vi "运维调试_总氮.vi"() -> ()   [LabVIEW 2016, in "斯坦道总氮.lvlib"]
uses:
  <vilib>/Utility/miscctls.llb/LVPointTypeDef.ctl
  <vilib>/Utility/config.llb/NI_LVConfig.lvlib
  <vilib>/ptbypt/NI_PtbyPt.lvlib
panel:
  out "固件版本号":string
  in  "定时设置":cluster{"启动":bool, "控制命令":T1, "测量参数":T2}(xcontrol)
  out "单位:":T3(ring)
  out "模块版本号":string
  in  "校准按钮":T4
  out "运行状态":T5 {"数据时间:" format="%<%y/%m/%d %H:%M:%S>T"; "仪器时间:" format="%<%y/%m/%d %H:%M:%S>T"}
  out "一级权限":bool
  out "二级权限":bool
  out "输入密码":u32
  out "布尔":bool
  in  "流程固件":bool
  in  "仪器参数设置":bool
  in  "量程参数读取":T6
  in  "模块启用":bool
  in  "串口设置":bool
  in  "公式一键写入":bool
  in  "流程路径":path=path "C:/Users/STD/Documents/斯坦道流程文件/流程.xml"
  in  "曲线模型":cluster{"X^2":dbl, "X":dbl, "B":dbl, "r^2":dbl}(xcontrol)
  out "字符串":string
  in  "质控参数设置":bool
  in  "自动测试量程配置":T7
  out "温度2":sgl
  out "温度1":sgl
  out "ADC":sgl
  in  "数组":string[](array[string])
  in  "量程切换阈值写入":bool
  in  "量程切换阈值读取":bool
  in  "参数下拉列表":enum16{"总磷", "总氮"}(ring)=enum."总氮"
  in  "量程下拉列表":enum16{"低量程", "高量程"}(ring)
  in  "测量模式下拉列表":enum16{"水样测量", "零点核查", "跨度核查", "标样核查", "加标回收"}(ring)
  in  "公式":cluster{"X^2":dbl, "X":dbl, "b":dbl}
  in  "写公式":bool
  in  "读公式":bool
  in  "返回":bool
  in  "设置":bool
  out "集成报警信息":string
  in  "停止":bool
  in  "手动启动":bool
  in  "单步测试":bool
  out "F3":sgl format="%#.6f"
  out "F2":sgl format="%#.6f"
  out "F1":sgl format="%#.6f"
  out "F0":sgl format="%#.6f"
  out "多列列表框":i32(listbox)
  # "参数设置"
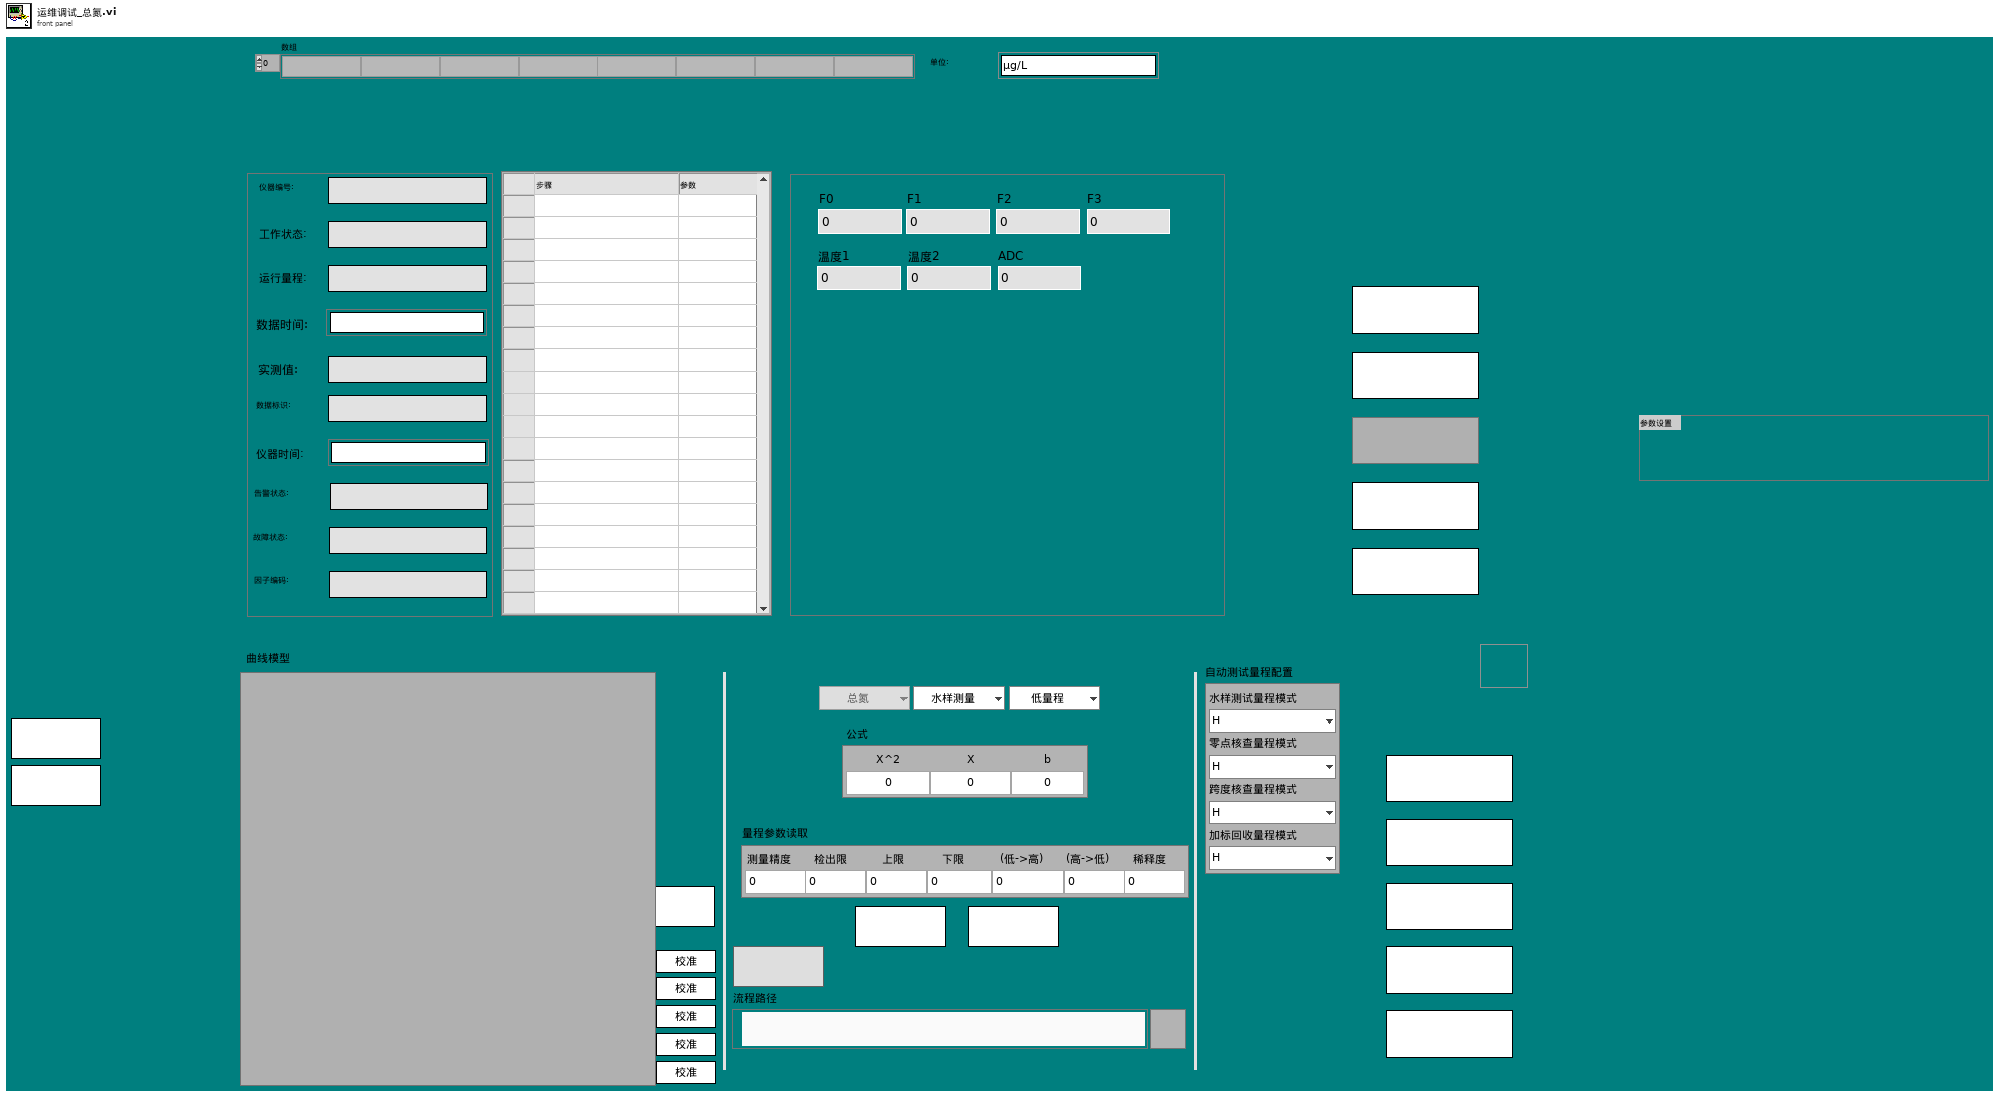
[diagram p1: front panel]
types:
  T1 = typedef "定时设置.xctl/国标控制命令.ctl" = enum16{"启动测量", "标样核查", "零点核查", "跨度核查", "空白测试", "平行样测试", "加标回收", "空白校准", "标样校准", "初始化（清洗）", "停止测试", "仪器重启", "校时", "模式设置", "测量间隔设置"}
  T2 = typedef "定时设置.xctl/测量参数.ctl" = u16
  T3 = enum16{"μg/L", "mg/L", "ppm", "mg/m3", "cm", "ppb", "μg/m3", "%", "nmol/mol", "μmol/mol", "MPN/L", "MPN/100ml", "ng/m3", "NTU", "无量纲", "mS/cm", "μS/cm", "℃", "mV", "cells/mL"}
  T4 = cluster{"校准1":bool, "校准2":bool, "校准3":bool, "校准4":bool, "校准5":bool}
  T5 = cluster{"仪器编号:":string, "工作状态:":string, "运行量程: ":string, "数据时间:":timestamp, "实测值:":string, "数据标识: ":string, "仪器时间:":timestamp, "告警状态: ":string, "故障状态:  ":string, "因子编码:":string}
  T6 = cluster{"测量精度":dbl, "检出限":dbl, "上限":dbl, "下限":dbl, "(低->高)":dbl, "(高->低)":dbl, "稀释度":dbl}
  T7 = cluster{"水样测试量程模式":enum16{"H", "L", "AUTO"}, "空白核查量程模式":enum16{"H", "L", "AUTO"}, "跨度核查量程模式":enum16{"H", "L", "AUTO"}, "加标回收量程模式":enum16{"H", "L", "AUTO"}}
  T8 = typedef "LVPointTypeDef.ctl" = cluster{"Horizontal":i16, "Vertical":i16}
  T9 = cluster{"因子编码":u32, "单位":u16, "标样参考值":sgl, "水样数据时间":timestamp, "水样实测值":sgl, "水样数据标识":string, "标样数据时间":timestamp, "标样实测值":sgl, "标样数据标识":string, "空白数据时间":timestamp, "空白实测值":sgl, "空白数据标识":string, "零点核查数据时间":timestamp, "零点核查实测值":sgl, "零点核查数据标识":string, "跨度核查数据时间":timestamp, "跨度核查实测值":sgl, "跨度核查数据标识":string, "加标回收数据时间":timestamp, "加标回收实测值":sgl, "加标回收数据标识":string, "平行样数据时间":timestamp, "平行样实测值":sgl, "平行样数据标识":string, "F0":sgl, "F1":sgl, "F2":sgl, "F3":sgl, "F4":sgl, "F5":sgl, "F6":sgl, "F7":sgl, "温度":sgl, "湿度":sgl, "X值":sgl, "fidrange":u16}
  T10 = cluster{"系统时间":timestamp, "工作状态":enum16{"空闲", "水样测试", "标样核查", "零点核查", "跨度核查", "空白测试", "平行样测试", "加标回收", "空白校准", "标样校准", "初始化（清洗）"}, "测量模式":enum16{"待机", "连续模式", "周期模式", "定点模式", "受控模式", "手动模式"}, "告警代码":u16, "故障代码":u16, "日志代码":u16, "软件版本":u16, "F0":sgl, "F1":sgl, "F2":sgl, "F3":sgl, "T":sgl, "H":sgl, "id":u16, "flowid":u16, "量程":u16, "总磷控温温度1":sgl, "营养盐控温温度2":sgl, "ADC":sgl}
  T11 = enum16{"空闲", "水样测试", "标样核查", "零点核查", "跨度核查", "空白测试", "平行样测试", "加标回收", "空白校准", "标样校准", "初始化（清洗）"}
  T12 = cluster{"Major":u16, "Minor":u16, "Fix":u16, "Build":u16}
  T13 = typedef "NI_LVConfig.lvlib/Config Data RefNum.ctl" = refnum<k1>
  T14 = cluster{"时间源选择":enum16{"系统时间源", "仪器时间源"}, "外部时间源":timestamp}
  T15 = enum32{"Bad", "Idle", "Run top level", "Running"}
  T16 = enum8{"Enabled", "Disabled", "Disabled and Grayed Out"}
  T17 = cluster{"运行模式":enum16{"维护模式", "常规模式", "应急模式", "质控模式"}, "质控频次":enum16{"关闭", "每天", "星期一", "星期二", "星期三", "星期四", "星期五", "星期六", "星期日"}, "空白核查时间":u16, "跨度核查时间":u16, "24H周期设置":bool[]}
  T18 = cluster{"时间标识":timestamp, "设备":string, "日志信息":string, "备注":string}
  T19 = cluster{"参数":string, "报警内容":string, "报警分析":string}
  T20 = cluster{"启动模式":enum16{"跨度核查", "水样测量", "空白核查", "标样核查", "加标回收"}, "启动参数":u16, "量程":enum16{"低量程", "高量程"}}
  T21 = cluster{"时间标识":timestamp, "设备":string, "日志信息":string, "流程参数":string}
  T22 = typedef "LVRowAndColumnUnsignedTypeDef.ctl" = cluster{"Row":u32, "Column":u32}
  T23 = cluster{"参数下拉列表":enum16{"总磷", "总氮"}, "测量模式下拉列表":enum16{"水样测量", "零点核查", "跨度核查", "标样核查", "加标回收"}, "量程下拉列表":enum16{"低量程", "高量程"}}
  T24 = cluster{"站号":u16, "量程切换":enum32{"H", "L", "AUTO"}, "控制命令":enum16{"启动测量", "标样核查", "零点核查", "跨度核查", "空白测试", "平行样测试", "加标回收", "空白校准", "标样校准", "初始化（清洗）", "停止测试", "仪器重启", "校时", "模式设置", "测量间隔设置"}, "模式设置":enum16{"待机", "连续模式", "周期模式", "定点模式", "受控模式", "手动模式"}, "测量间隔":u16}
  T25 = cluster{"跨度值":dbl, "零点标准液浓度":dbl, "跨度标准液浓度":dbl, "标准液标准浓度":dbl}
  T26 = cluster{"确定":bool, "跨度值":dbl, "零点标准液浓度":dbl, "跨度标准液浓度":dbl, "标准液标准浓度":dbl}
  T27 = cluster{"测量量程":dbl, "测量精度":dbl, "测量间隔":dbl, "消解温度":dbl, "消解时长":dbl, "空白校准时间":timestamp, "曲线截距":dbl, "曲线斜率":dbl, "测量检出限":dbl, "测量信号值":dbl, "线性相关系数":dbl, "二次多项式系数":dbl, "标样校准时间":timestamp, "稀释倍数":dbl, "三项式系数":dbl, "空白标定系数":dbl, "量程系数":dbl, "F0/ORPA":dbl, "F1/ORPB":dbl, "F2/ORPK":dbl, "F3":dbl, "F4":dbl, "F5":dbl, "F6":dbl, "F7":dbl, "X0/滴定数":dbl, "量程":dbl}
  T28 = cluster{"确定":bool, "测量量程":dbl, "测量精度":dbl, "测量间隔":dbl, "消解温度":dbl, "消解时长":dbl, "空白校准时间":timestamp, "曲线截距":dbl, "曲线斜率":dbl, "测量检出限":dbl, "测量信号值":dbl, "线性相关系数":dbl, "二次多项式系数":dbl, "标样校准时间":timestamp, "稀释倍数":dbl, "三项式系数":dbl, "空白标定系数":dbl, "量程系数":dbl, "F0/ORPA":dbl, "F1/ORPB":dbl, "F2/ORPK":dbl, "F3":dbl, "F4":dbl, "F5":dbl, "F6":dbl, "F7":dbl, "X0/滴定数":dbl, "量程":dbl}
  T29 = cluster{"标液浓度1":dbl, "标液浓度2":dbl, "标液浓度3":dbl, "标液浓度4":dbl, "标液浓度5":dbl}
  T30 = cluster{"测量精度":u16, "检出限":dbl, "上限":dbl, "下限":dbl, "阈值（低->高）":dbl, "阈值（高->低）":dbl, "稀释度":dbl}
  T31 = enum16{"Left Button", "Center Button", "Right Button", "Window Close"}
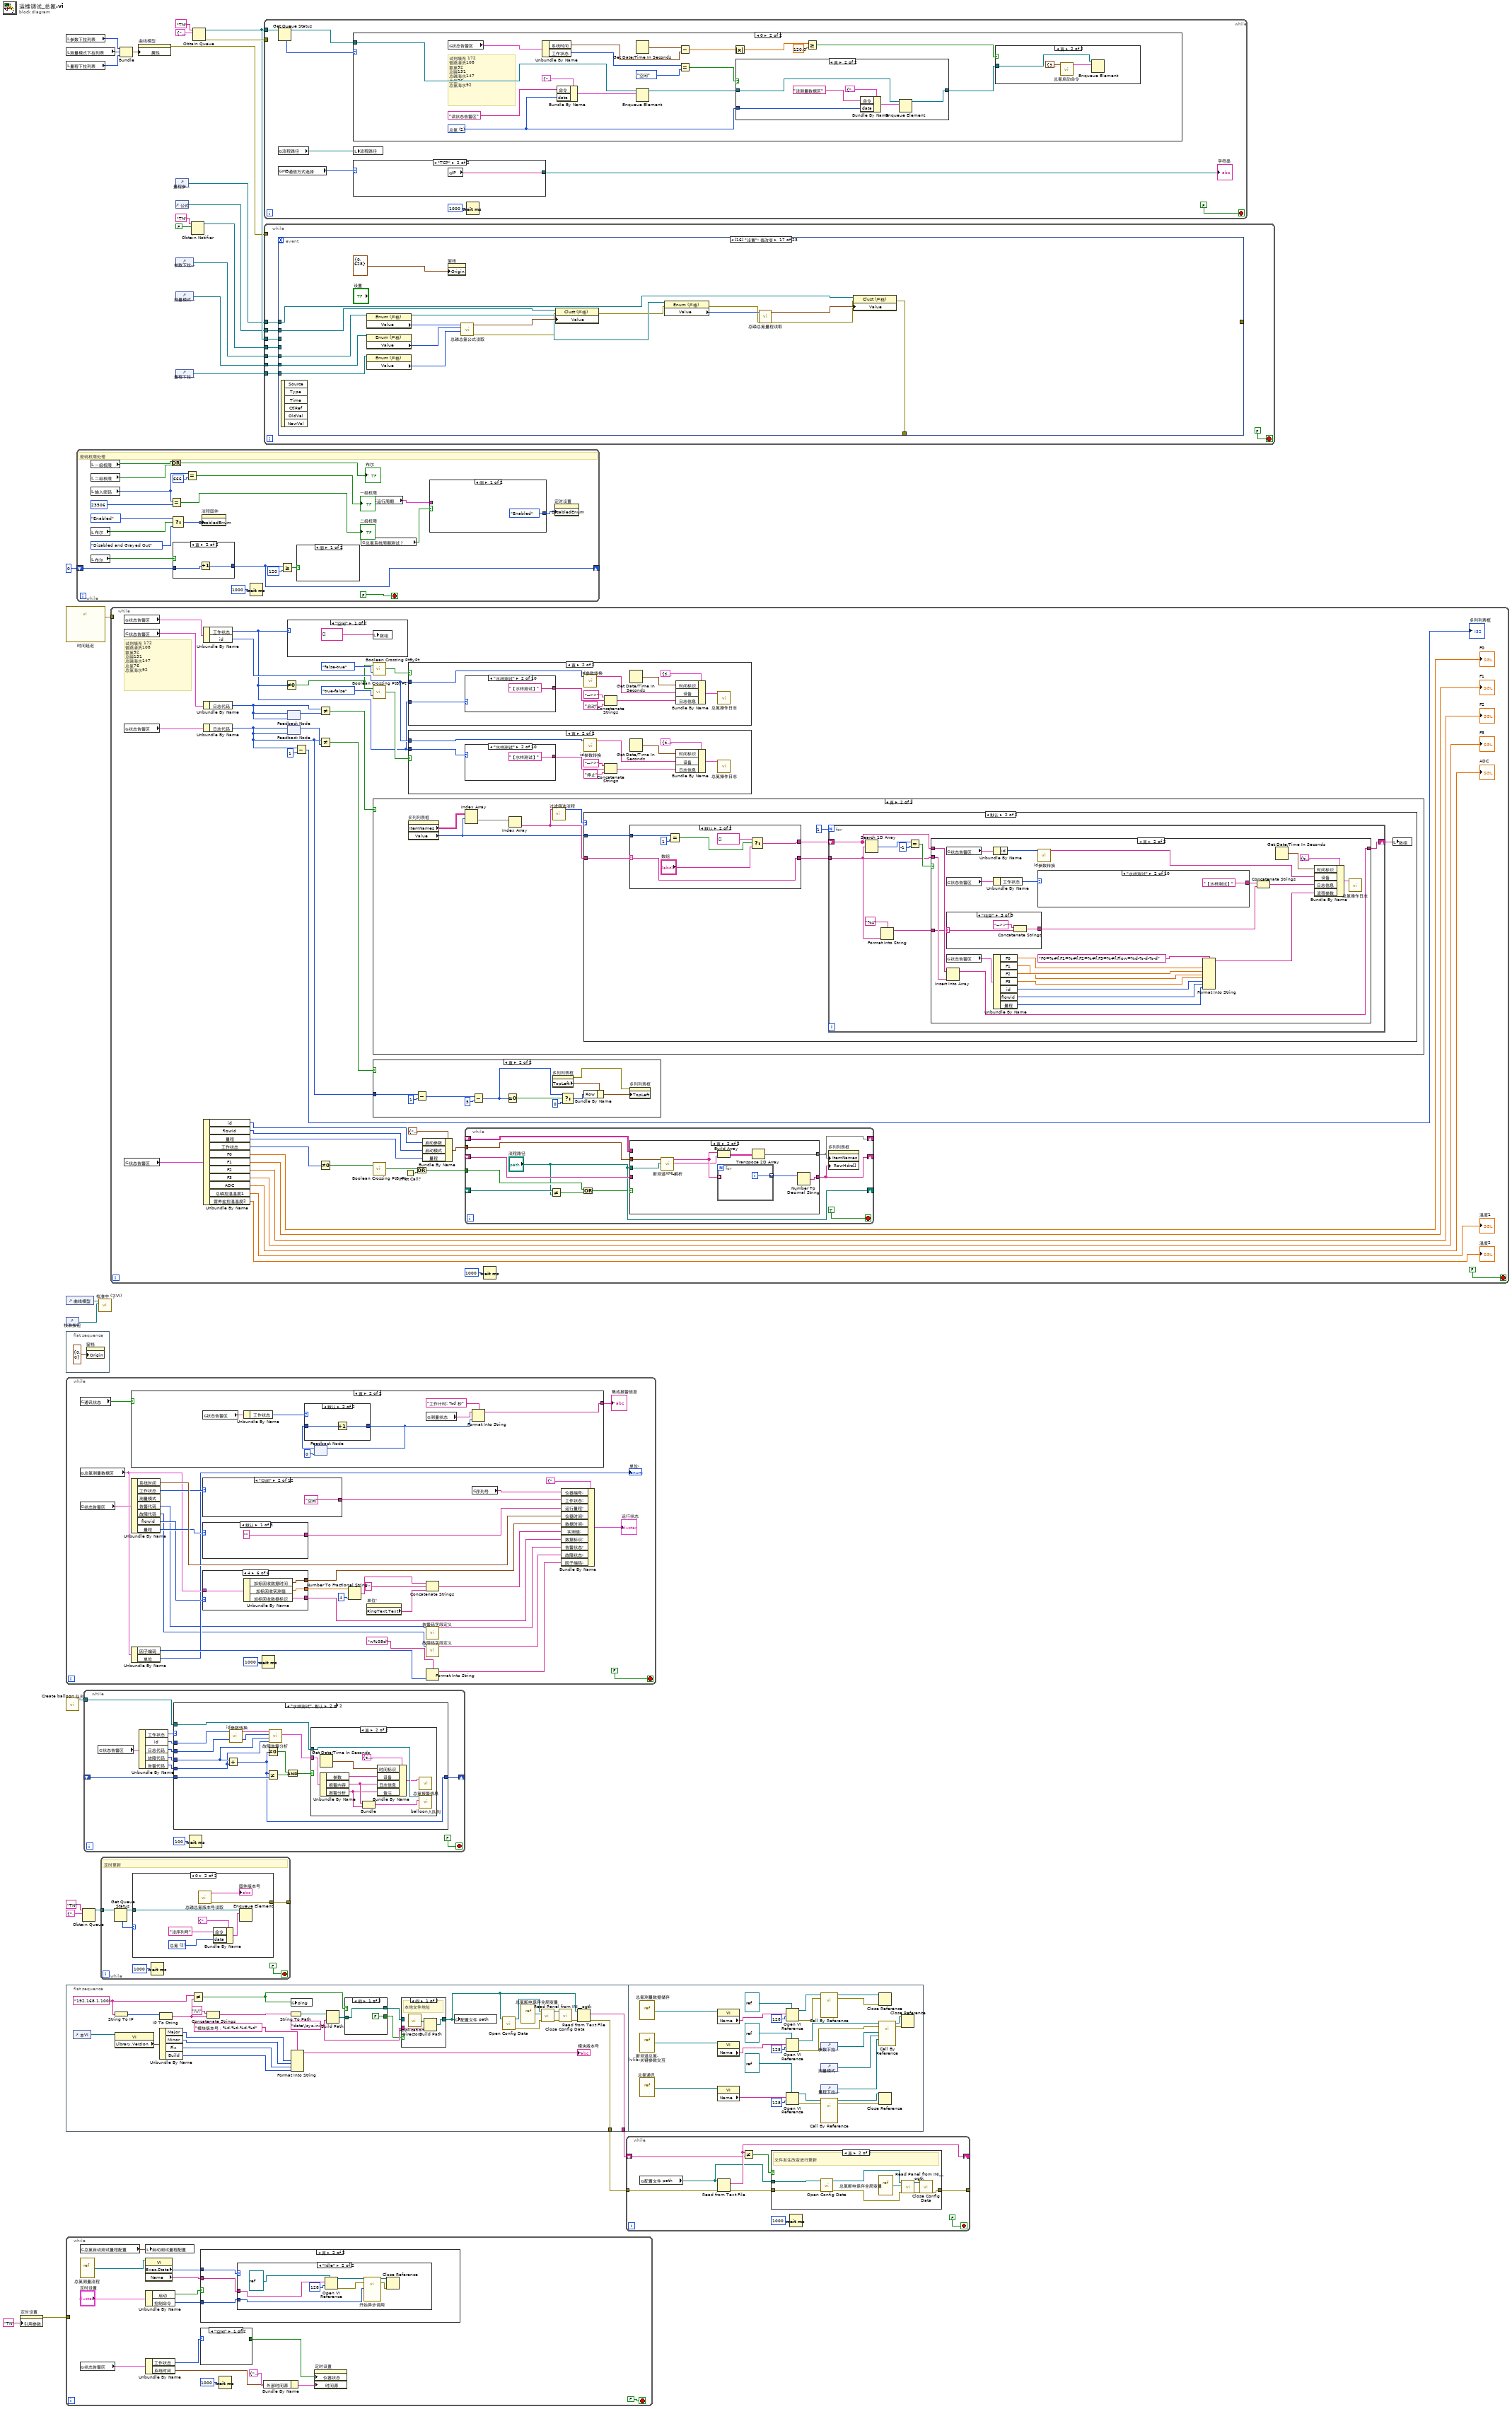
[diagram p0: block diagram]
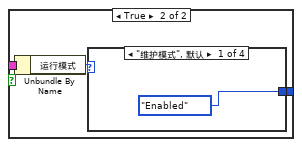
[diagram p5: hidden frame]
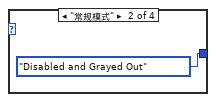
[diagram p6: hidden frame]
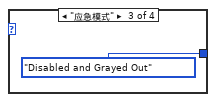
[diagram p7: hidden frame]
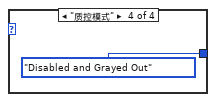
[diagram p8: hidden frame]
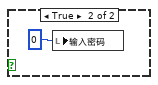
[diagram p9: hidden frame]
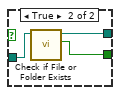
[diagram p11: hidden frame]
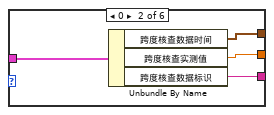
[diagram p15: hidden frame]
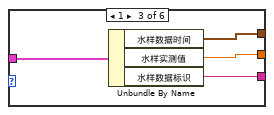
[diagram p16: hidden frame]
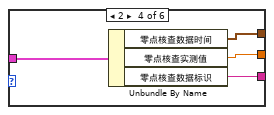
[diagram p17: hidden frame]
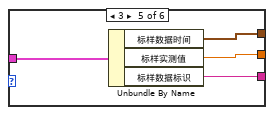
[diagram p18: hidden frame]
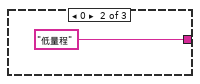
[diagram p19: hidden frame]
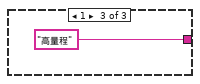
[diagram p20: hidden frame]
diagram:
  n1 = property on="定时设置" class="定时设置 (严格)"("引用参数"="TN") -> (error out=w1:errorcluster)  [unwired: 2 in, 1 out]
  n2 = local read "参数下拉列表"() -> (w12:enum16{"总磷", "总氮"})
  n3 = local read "测量模式下拉列表"() -> (w11:enum16{"水样测量", "零点核查", "跨度核查", "标样核查", "加标回收"})
  n4 = local read "量程下拉列表"() -> (w10:enum16{"低量程", "高量程"})
  n5 = call "时间延迟"() -> ("error out"=w21:errorcluster)  [unwired: 11 in]
  n6 = control-ref of="曲线模型"() -> (w6:refnum<vi>)
  n7 = control-ref of="校准按钮"() -> (w5:refnum<vi>)
  n8 = flat-sequence {
    frame #0 {
      n9 = property on="窗格" class="Pane"("Origin"=T8 {"Horizontal"=0, "Vertical"=0} ("原点")) -> ()  [unwired: 2 in, 2 out]
    }
  }
  n10 = while {
    stop <- FALSE stop-if-true
    n11 = global read "VAR总氮全局变量.vi" "通讯状态"() -> (w59:bool)
    n12 = global read "VAR总氮全局变量.vi" "总氮测量数据区"() -> (w48:T9)
    n13 = global read "VAR总氮全局变量.vi" "状态告警区"() -> (w51:T10)
    n14 = case shown="真" w59 {
      tunnel: ["通讯异常" ("集成报警信息") w102] -> w58
      frame False {
      }
      frame True {
        n15 = global read "VAR总氮全局变量.vi" "状态告警区"() -> (w108:T10)
        n16 = Unbundle By Name(w108) -> ("工作状态"=w107:T11)
        n17 = feedback #1(0) -> (w105:i32)
        n18 = case shown="默认" w107 {
          tunnel: w105 -> [_ w110]
          tunnel: [_ w109] -> w103
          frame "空闲" {
          }
          frame Default {
            n19 = Increment(x=w110) -> (x+1=w109:i32)
          }
        }
        n20 = feedback-in #1(w103) -> ()
        n21 = global read "VAR总氮全局变量.vi" "测量状态"() -> (w101:string)
        n22 = Format Into String(format string="工作计时: %d 秒" ("格式字符串"), initial string=w101, w103) -> (resulting string=w102:string)  [unwired: 1 in, 1 out]
      }
    }
    "集成报警信息" <- w58
    n23 = Unbundle By Name(w51) -> ("系统时间"=w57:timestamp, "工作状态"=w49:T11, "告警代码"=w34:u16, "故障代码"=w32:u16, "flowid"=w47:u16, "量程"=w55:u16)  [unwired: 1 out]
    n24 = Unbundle By Name(w48) -> ("因子编码"=w52:u32, "单位"=→"单位:":u16)
    n25 = case shown="\"空闲\"" w49 {
      selector: w49 -> [w85 _ _ _ _ _ _ _ _ _ _ _]
      tunnel: [w86 "空闲" ("工作状态") "水样测量" ("工作状态") "标样核查" ("工作状态") "零点核查" ("工作状态") "跨度核查" ("工作状态") "空白测试" ("工作状态") "平行样测试" ("工作状态") "加标回收" ("工作状态") "空白校准" ("工作状态") "标样校准" ("工作状态") "初始化" ("工作状态")] -> w56
      frame Default {
        n26 = Format Into String(format string="%d" ("格式字符串"), initial string="未知" ("工作状态"), w85) -> (resulting string=w86:string)  [unwired: 1 in, 1 out]
      }
      frame "空闲" {
      }
      frame "水样测试" {
      }
      frame "标样核查" {
      }
      frame "零点核查" {
      }
      frame "跨度核查" {
      }
      frame "空白测试" {
      }
      frame "平行样测试" {
      }
      frame "加标回收" {
      }
      frame "空白校准" {
      }
      frame "标样校准" {
      }
      frame "初始化（清洗）" {
      }
    }
    n27 = case shown="默认" w55 {
      tunnel: ["" ("字符串") "低量程" ("字符串") "高量程" ("字符串")] -> w54
      frame Default {
      }
      frame 0 {
      }
      frame 1 {
      }
    }
    n28 = case shown="4" w47 {
      tunnel: [_ w65 w69 w73 w77 w81] -> w43
      tunnel: [_ w63 w68 w72 w76 w80] -> w39
      tunnel: [_ w62 w67 w71 w75 w79] -> w36
      tunnel: w48 -> [_ w64 w66 w70 w74 w78]
      frame Default {
      }
      frame 0 {
        n29 = Unbundle By Name(w64) -> ("跨度核查数据时间"=w65:timestamp, "跨度核查实测值"=w63:sgl, "跨度核查数据标识"=w62:string)
      }
      frame 1 {
        n30 = Unbundle By Name(w66) -> ("水样数据时间"=w69:timestamp, "水样实测值"=w68:sgl, "水样数据标识"=w67:string)
      }
      frame 2 {
        n31 = Unbundle By Name(w70) -> ("零点核查数据时间"=w73:timestamp, "零点核查实测值"=w72:sgl, "零点核查数据标识"=w71:string)
      }
      frame 3 {
        n32 = Unbundle By Name(w74) -> ("标样数据时间"=w77:timestamp, "标样实测值"=w76:sgl, "标样数据标识"=w75:string)
      }
      frame 4 {
        n33 = Unbundle By Name(w78) -> ("加标回收数据时间"=w81:timestamp, "加标回收实测值"=w80:sgl, "加标回收数据标识"=w79:string)
      }
    }
    n34 = Wait (ms)(milliseconds to wait=u32 1000 ("等待时间（毫秒）")) -> ()  [unwired: 1 out]
    n35 = Number To Fractional String(number=w39, precision (6)=i16 4 ("精度(6)")) -> (F-format string=w38:string)  [unwired: 2 in]
    n36 = property on="单位:" class="Enum (严格)"() -> ("RingText.Text"=w40:string)  [unwired: 2 in, 2 out]
    n37 = Concatenate Strings(w38, " " ("字符串"), w40) -> (w37:string)
    n38 = call "告警码字段定义.vi"("告警代码"=w34) -> ("字符串"=w33:string)  [unwired: 8 in, 2 out]
    n39 = call "故障码字段定义.vi"("故障代码"=w32) -> ("字符串"=w31:string)  [unwired: 10 in]
    n40 = Format Into String(format string="w%05d" ("格式字符串"), w52) -> (resulting string=w35:string)  [unwired: 2 in, 1 out]
    n41 = global read "VAR总氮全局变量.vi" "序列号"() -> (w50:string)
    n42 = Bundle By Name(cluster=T5 {"仪器编号:"="", "工作状态:"="", "运行量程: "="", "数据时间:"=timestamp(0 s since 1904-01-01), "实测值:"="", "数据标识: "="", "仪器时间:"=timestamp(0 s since 1904-01-01), "告警状态: "="", "故障状态:  "="", "因子编码:"=""} ("运行状态"), "仪器编号:"=w50, "工作状态:"=w56, "运行量程:"=w54, "仪器时间:"=w57, "数据时间:"=w43, "实测值:"=w37, "数据标识:"=w36, "告警状态:"=w33, "故障状态:"=w31, "因子编码:"=w35) -> (→"运行状态":T5)
  }
  n43 = call "Create balloon 队列.vi"() -> ("队列输出"=w3:refnum<queue>)  [unwired: 11 in]
  n44 = flat-sequence {
    tunnel: [w120] -> w4
    tunnel: [w119] -> w7
    frame #0 {
      w133 = "data\\sys.ini" ("名称或相对路径")
      w125 = "192.168.1.100" ("名称")
      n45 = control-ref of="本VI"() -> (w118:refnum<vi>)
      n46 = String To IP(1:w125) -> (0:w132:u32)
      n47 = property class="VI"(reference=w118) -> ("Library.Version"=w117:T12)  [unwired: 1 in, 2 out]
      n48 = IP To String(2:w132) -> (0:w129:string)  [unwired: 1 in]
      n49 = Unbundle By Name(w117) -> ("Major"=w115:u16, "Minor"=w114:u16, "Fix"=w113:u16, "Build"=w112:u16)
      n50 = Not Equal?(x=w125, y=w129) -> (x != y?=w123:bool)
      n51 = Concatenate Strings("\\\\" ("字符串"), w129) -> (w130:string)
      n52 = String To Path(string=w130) -> (path=w124:path)
      n53 = global write "VAR总氮全局变量.vi" "ping"(w123) -> ()
      n54 = Format Into String(format string="模块版本号：%d.%d.%d.%d" ("格式字符串"), w115, w114, w113, w112) -> (resulting string=→"模块版本号":string)  [unwired: 2 in, 1 out]
      n55 = Build Path(base path=w124, name or relative path=w133) -> (appended path=w128:path)
      n56 = case shown="假" w123 {
        tunnel: w128 -> [w139 w143]
        tunnel: [w139 w142] -> w127
        tunnel: [FALSE w141] -> w126
        frame False {
        }
        frame True {
          n57 = call <vilib>:"Check if File or Folder Exists.vi"("path"=w143) -> ("file or folder exists?"=w141:bool, "dup path"=w142:path)  [unwired: 8 in, 1 out]
        }
      }
      n58 = case shown="假" w126 {
        tunnel: w127 -> [_ w147]
        tunnel: [w145 w147] -> w122
        tunnel: w133 -> [w144 _]
        frame False {
          # "本地文件地址"
          n59 = call <vilib>:"Application Directory.vi"() -> ("Application Directory"=w146:path)
          n60 = Build Path(base path=w146, name or relative path=w144) -> (appended path=w145:path)
        }
        frame True {
          # "网络共享地址"
        }
      }
      n61 = global write "VAR总氮全局变量.vi" "配置文件 path"(w122) -> ()
      n62 = call <vilib>:"Open Config Data.vi"("configuration file path"=w122) -> ("error out"=w135:errorcluster, "refnum"=w138:T13)  [unwired: 8 in, 1 out]
      n63 = vi-ref "总氮断电保存全局变量.vi"() -> (w137:refnum<vi>)
      n64 = call <userlib>:"Read Panel from INI__ogtk.vi"("error in (no error)"=w135, "VI ref"=w137, "refnum"=w138) -> ("error out"=w134:errorcluster, "refnum out"=w136:T13)  [unwired: 7 in]
      n65 = call <vilib>:"Close Config Data.vi"("error in (no error)"=w134, "refnum"=w136) -> ("error out"=w121:errorcluster)  [unwired: 8 in, 1 out]
      n66 = Read from Text File(file (use dialog)=w122, error in=w121) -> (text=w119:string, error out=w120:errorcluster)  [unwired: 2 in, 2 out]
    }
    frame #1 {
      n67 = vi-ref "总氮测量数据储存.vi"() -> (w166:refnum<vi>)
      n68 = vi-ref "斯坦道总氮.lvlib:关键参数交互.vi"() -> (w151:refnum<vi>)
      n69 = vi-ref "总氮通讯.vi"() -> (w174:refnum<vi>)
      n70 = property class="VI"(reference=w166) -> ("Name"=w159:string)  [unwired: 1 in, 2 out]
      n71 = property class="VI"(reference=w151) -> ("Name"=w158:string)  [unwired: 1 in, 2 out]
      n72 = property class="VI"(reference=w174) -> ("Name"=w173:string)  [unwired: 1 in, 2 out]
      n73 = Open VI Reference(type specifier VI Refnum (for type only)=refnum<vi> refnum, vi path=w159, options=128 ("选项")) -> (vi reference=w161:refnum<vi>, error out=w163:errorcluster)  [unwired: 3 in]
      n74 = Open VI Reference(type specifier VI Refnum (for type only)=refnum<vi> refnum, vi path=w158, options=128 ("选项")) -> (vi reference=w156:refnum<vi>, error out=w154:errorcluster)  [unwired: 3 in]
      n75 = Open VI Reference(type specifier VI Refnum (for type only)=refnum<vi> refnum, vi path=w173, options=128 ("选项")) -> (vi reference=w171:refnum<vi>, error out=w169:errorcluster)  [unwired: 3 in]
      n76 = call-by-ref "?"(reference=w161, error in=w163) -> (reference out=w165:refnum<vi>, error out=w164:errorcluster)  [unwired: 12 in]
      n77 = control-ref of="参数下拉列表"() -> (w150:refnum<vi>)
      n78 = control-ref of="测量模式下拉列表"() -> (w149:refnum<vi>)
      n79 = control-ref of="量程下拉列表"() -> (w148:refnum<vi>)
      n80 = call-by-ref "?"(reference=w171, error in=w169) -> (reference out=w167:refnum<vi>, error out=w168:errorcluster)  [unwired: 12 in]
      n81 = Close Reference(reference=w165, error in (no error)=w164) -> ()  [unwired: 1 out]
      n82 = call-by-ref "?"(reference=w156, error in=w154, "量程下拉列表"=w148, "测量模式下拉列表"=w149, "测量参数"=w150) -> (reference out=w152:refnum<vi>, error out=w153:errorcluster)  [unwired: 9 in]
      n83 = Close Reference(reference=w167, error in (no error)=w168) -> ()  [unwired: 1 out]
      n84 = Close Reference(reference=w152, error in (no error)=w153) -> ()  [unwired: 1 out]
    }
  }
  n85 = while {
    tunnel: w1 -> [_]
    stop <- FALSE stop-if-true
    n86 = global read "总氮断电保存全局变量.vi" "总氮自动测试量程配置"() -> (w187:T7)
    n87 = vi-ref "总氮测量流程.vi"() -> (w186:refnum<vi>)
    n88 = global read "VAR总氮全局变量.vi" "状态告警区"() -> (w180:T10)
    n89 = local write "自动测试量程配置"(w187) -> ()
    n90 = property class="VI"(reference=w186) -> ("Exec.State"=w184:T15, "Name"=w185:string)  [unwired: 1 in, 2 out]
    n91 = Unbundle By Name("定时设置") -> ("启动"=w181:bool, "控制命令"=w182:T1)
    n92 = Unbundle By Name(w180) -> ("工作状态"=w179:T11, "系统时间"=w175:timestamp)
    n93 = case shown="真" w181 {
      tunnel: w185 -> [_ w193]
      tunnel: w182 -> [_ w192]
      tunnel: w184 -> [_ w191]
      frame False {
      }
      frame True {
        n94 = case shown="\"Idle\"" w191 {
          tunnel: w193 -> [_ w197]
          tunnel: w192 -> [_ w195]
          frame "Bad", Default {
          }
          frame "Idle" {
            n95 = Open VI Reference(type specifier VI Refnum (for type only)=refnum<vi> refnum, vi path=w197, options=128 ("选项")) -> (vi reference=w198:refnum<vi>, error out=w199:errorcluster)  [unwired: 3 in]
            n96 = call-by-ref "开始异步调用"(reference=w198, error in=w199, "控制命令"=w195) -> (reference out=w200:refnum<vi>, error out=w201:errorcluster)  [unwired: 11 in]
            n97 = Close Reference(reference=w200, error in (no error)=w201) -> ()  [unwired: 1 out]
          }
        }
      }
    }
    n98 = case shown="\"空闲\"" w179 {
      tunnel: [_ TRUE] -> w178
      frame "空闲" {
      }
      frame "水样测试", Default {
      }
    }
    n99 = Wait (ms)(milliseconds to wait=u32 1000 ("等待时间（毫秒）")) -> ()  [unwired: 1 out]
    n100 = Bundle By Name(cluster=T14 {"时间源选择"=enum."仪器时间源", "外部时间源"=timestamp(0 s since 1904-01-01)} ("时间源"), "外部时间源"=w175) -> (w176:T14)
    n101 = property on="定时设置" class="定时设置 (严格)"("仪器状态"=w178, "时间源"=w176) -> ()  [unwired: 2 in, 2 out]
  }
  n102 = while {
    shift-right: [w211] -> _
    shift-left: u32 0 ("等待时间（毫秒）") -> [w212]
    stop <- FALSE stop-if-true
    # "密码权限处理"
    n103 = local read "一级权限"() -> (w215:bool)
    n104 = local read "二级权限"() -> (w216:bool)
    n105 = local read "输入密码"() -> (w219:u32)
    n106 = local read "布尔"() -> (w208:bool)
    n107 = local read "布尔"() -> (w213:bool)
    n108 = Or(x=w215, y=w216) -> (x .or. y?=→"布尔":bool)
    n109 = Equal?(x=w219, y=u32 23506) -> (x = y?=→"二级权限":bool)
    n110 = Select(t=T16."Enabled" ("禁用"), s=w208, f=T16."Disabled and Grayed Out") -> (s? t:f=w206:T16)
    n111 = case shown="真" w213 {
      tunnel: w212 -> [_ w234]
      tunnel: [_ w233] -> w211
      frame False {
      }
      frame True {
        n112 = Increment(x=w234) -> (x+1=w233:u32)
      }
    }
    n113 = Equal?(x=w219, y=u32 666) -> (x = y?=→"一级权限":bool)
    n114 = property on="流程固件" class="Bool"("DisabledEnum"=w206) -> ()  [unwired: 2 in, 2 out]
    n115 = Wait (ms)(milliseconds to wait=u32 1000 ("等待时间（毫秒）")) -> ()  [unwired: 1 out]
    n116 = Greater Or Equal?(x=w211, y=u32 120) -> (x >= y?=w209:bool)
    n117 = case shown="假" w209 {
      frame False {
      }
      frame True {
        n118 = local write "输入密码"(u32 0 ("输入密码")) -> ()
      }
    }
    n119 = global read "总氮断电保存全局变量.vi" "总氮系统周期测试？"() -> (w203:bool)
    n120 = global read "总氮断电保存全局变量.vi" "运行周期"() -> (w204:T17)
    n121 = case shown="假" w203 {
      tunnel: w204 -> [_ w227]
      tunnel: [T16."Enabled" ("禁用") w225] -> w202
      frame False {
      }
      frame True {
        n122 = Unbundle By Name(w227) -> ("运行模式"=w226:enum16{"维护模式", "常规模式", "应急模式", "质控模式"})
        n123 = case shown="\"维护模式\", 默认" w226 {
          tunnel: [T16."Enabled" ("禁用") T16."Disabled and Grayed Out" ("禁用") T16."Disabled and Grayed Out" ("禁用") T16."Disabled and Grayed Out" ("禁用")] -> w225
          frame "维护模式", Default {
          }
          frame "常规模式" {
          }
          frame "应急模式" {
          }
          frame "质控模式" {
          }
        }
      }
    }
    n124 = property on="定时设置" class="定时设置 (严格)"("DisabledEnum"=w202) -> ()  [unwired: 2 in, 2 out]
  }
  n125 = Obtain Queue(name (unnamed)="TN" ("名称（未命名）"), element data type=cluster{"命令":string, "data":variant} {"命令"="", "data"=variant}) -> (queue out=w18:refnum<queue>)  [unwired: 3 in, 2 out]
  n126 = while {
    tunnel: w3 -> [w241]
    shift-right: [w237] -> _
    shift-left: _ -> [w238]
    stop <- FALSE stop-if-true
    n127 = global read "VAR总氮全局变量.vi" "状态告警区"() -> (w235:T10)
    n128 = Unbundle By Name(w235) -> ("工作状态"=w236:T11, "id"=w243:u16, "日志代码"=w242:u16, "故障代码"=w240:u16, "告警代码"=w239:u16)
    n129 = case shown="\"水样测试\", 默认" w236 {
      tunnel: w243 -> [_ w258]
      tunnel: w242 -> [_ w257]
      tunnel: w241 -> [_ w254]
      tunnel: w240 -> [_ w253]
      tunnel: w239 -> [_ w252]
      tunnel: w238 -> [w246 w251]
      tunnel: [w246 w250] -> w237
      frame "空闲" {
      }
      frame "水样测试", Default {
        n130 = Add(x=w253, y=w252) -> (x+y=w250:u16)
        n131 = call "id参数转换.vi"("id"=w258) -> ("table输出"=w255:string)  [unwired: 10 in]
        n132 = Not Equal To 0?(x=w250) -> (x != 0?=w249:bool)
        n133 = Not Equal?(x=w250, y=w251) -> (x != y?=w248:bool)
        n134 = call "故障告警分析.vi"("告警代码"=w252, "故障代码"=w253, "运行步序"=w257, "参数"=w255) -> ("报警内容"=w256:T19)  [unwired: 6 in, 1 out]
        n135 = And(x=w249, y=w248) -> (x .and. y?=w247:bool)
        n136 = case shown="真" w247 {
          tunnel: w256 -> [_ w267]
          tunnel: w254 -> [_ w266]
          frame False {
          }
          frame True {
            n137 = Get Date/Time In Seconds() -> (seconds since 1Jan1904=w265:timestamp)
            n138 = Unbundle By Name(w267) -> ("参数"=w262:string, "报警内容"=w261:string, "报警分析"=w260:string)
            n139 = Bundle("报警内容"=w261, "报警分析"=w260) -> (w259:cluster{"报警内容":string, "报警分析":string})  [unwired: 1 in]
            n140 = Bundle By Name(cluster=T18 {"时间标识"=timestamp(0 s since 1904-01-01), "设备"="", "日志信息"="", "备注"=""} ("data in"), "时间标识"=w265, "设备"=w262, "日志信息"=w261, "备注"=w260) -> (w264:T18)
            n141 = call "总氮报警信息.vi"("data in"=w264) -> ()  [unwired: 10 in, 1 out]
            n142 = call "balloon入队列.vi"("报警内容"=w259, "队列"=w266) -> ()  [unwired: 9 in, 1 out]
          }
        }
      }
    }
    n143 = Wait (ms)(milliseconds to wait=u32 100) -> ()  [unwired: 1 out]
  }
  n144 = call "校准中 (子VI).vi"("曲线模型"=w6, "校准按钮"=w5) -> ()  [unwired: 9 in]
  n145 = while {
    tunnel: w18 -> [w272]
    tunnel: [w270] -> _
    stop <- FALSE stop-if-true
    # "定时更新"
    n146 = Get Queue Status(queue=w272) -> (queue out=w269:refnum<queue>, # elements in queue=w268:i32)  [unwired: 2 in, 6 out]
    n147 = case shown="0" w268 {
      tunnel: [_ w276] -> w270
      tunnel: w269 -> [_ w275]
      frame Default {
      }
      frame 0 {
        w278 = u16 2 items=["总磷"=1, "总氮"=2, "氨氮"=3] ("站号")
        n148 = call "总磷总氮版本号读取.vi"() -> ("error out"=w276:errorcluster, "固件版本号"=→"固件版本号":string)  [unwired: 10 in]
        n149 = Bundle By Name(cluster=cluster{"命令":string, "data":variant} {"命令"="", "data"=variant} ("元素"), "命令"="读序列号", "data"=w278) -> (w277:cluster{"命令":string, "data":variant})
        n150 = Enqueue Element(queue=w275, element=w277) -> ()  [unwired: 2 in, 3 out]
      }
    }
    n151 = Wait (ms)(milliseconds to wait=u32 1000 ("等待时间（毫秒）")) -> ()  [unwired: 1 out]
  }
  n152 = while {
    tunnel: w21 -> [_]
    stop <- FALSE stop-if-true
    # "试剂填充 172 \n管路清洗108\n氨氮92\n总磷131\n总磷海水147\n总氮76\n总氮海水92"
    n153 = global read "VAR总氮全局变量.vi" "状态告警区"() -> (w301:T10)
    n154 = global read "VAR总氮全局变量.vi" "状态告警区"() -> (w299:T10)
    n155 = global read "VAR总氮全局变量.vi" "状态告警区"() -> (w303:T10)
    n156 = global read "VAR总氮全局变量.vi" "状态告警区"() -> (w311:T10)
    n157 = Unbundle By Name(w301) -> ("工作状态"=w281:T11, "id"=w285:u16)
    n158 = Unbundle By Name(w299) -> ("日志代码"=w298:u16)
    n159 = Unbundle By Name(w303) -> ("日志代码"=w295:u16)
    n160 = Unbundle By Name(w311) -> ("id"=w308:u16, "flowid"=w310:u16, "量程"=w309:u16, "工作状态"=w289:T11, "F0"=→"F0":sgl, "F1"=→"F1":sgl, "F2"=→"F2":sgl, "F3"=→"F3":sgl, "ADC"=→"ADC":sgl, "总磷控温温度1"=→"温度1":sgl, "营养盐控温温度2"=→"温度2":sgl)
    n161 = Not Equal To 0?(x=w281) -> (x != 0?=w283:bool)
    n162 = case shown="\"空闲\"" w281 {
      frame "空闲" {
        n163 = local write "数组"(string[] [] ("数组")) -> ()
      }
      frame "水样测试", Default {
      }
    }
    n164 = feedback #2(w298) -> (w300:u16)
    n165 = feedback-in #2(w298) -> ()
    n166 = feedback-in #3(w295) -> ()
    n167 = feedback #3(w295) -> (w316:u16)
    n168 = Subtract(x=w295, y=1) -> (x-y=→"多列列表框":i32)
    n169 = Not Equal?(x=w298, y=w300) -> (x != y?=w297:bool)
    n170 = Not Equal?(x=w295, y=w316) -> (x != y?=w315:bool)
    n171 = Not Equal To 0?(x=w289) -> (x != 0?=w313:bool)
    n172 = call <vilib>:"Boolean Crossing PtByPt.vi"("direction"=enum16{"either", "false-true", "true-false"}."false-true", "input"=w283) -> ("crossing"=w287:bool)  [unwired: 1 in]
    n173 = call <vilib>:"Boolean Crossing PtByPt.vi"("direction"=enum16{"either", "false-true", "true-false"}."true-false", "input"=w283) -> ("crossing"=w282:bool)  [unwired: 1 in]
    n174 = case shown="真" w297 {
      frame False {
      }
      frame True {
        n175 = property on="多列列表框" class="MCListbox (严格)"() -> ("ItemNames"=w362:string[][], "Value"=w358:i32)  [unwired: 2 in, 2 out]
        n176 = Index Array(array=w362, index (row)=w358) -> (element=w361:string[])  [unwired: 1 in]
        n177 = Index Array(array=w361) -> (element=w360:string)  [unwired: 1 in]
        n178 = call "过滤筛选流程.vi"("字符串"=w360) -> ("匹配后偏移量"=w359:i32)  [unwired: 10 in]
        n179 = case shown="默认" w359 {
          tunnel: w360 -> [_ w364]
          tunnel: w358 -> [_ w363]
          frame -1 {
          }
          frame Default {
            n180 = case shown="默认" w364 {
              selector: w364 -> [w370 w377]
              tunnel: [w370 w377] -> w366
              tunnel: [string[] [] ("数组") w372] -> w365
              tunnel: w363 -> [_ w376]
              frame "读数" {
              }
              frame Default {
                n181 = Equal?(x=w376, y=1) -> (x = y?=w374:bool)
                n182 = Select(t=string[] [], s=w374, f="数组") -> (s? t:f=w372:string[])
              }
            }
            n183 = for {
              N: 1 -> [_]
              tunnel: w366 -> [w379]
              shift-right: [w378] -> w367
              shift-left: w365 -> [w380]
              n184 = Search 1D Array(1D array=w380, element=w379) -> (index of element=w383:i32)  [unwired: 1 in]
              n185 = Format Into String(format string="%s" ("格式字符串"), w379) -> (resulting string=w384:string)  [unwired: 2 in, 1 out]
              n186 = Equal?(x=w383, y=-1) -> (x = y?=w381:bool)
              n187 = case shown="真" w381 {
                tunnel: w384 -> [_ w394]
                tunnel: w380 -> [w386 w398]
                tunnel: w379 -> [_ w397]
                tunnel: [w386 w396] -> w378
                frame False {
                }
                frame True {
                  n188 = global read "VAR总氮全局变量.vi" "状态告警区"() -> (w411:T10)
                  n189 = global read "VAR总氮全局变量.vi" "状态告警区"() -> (w393:T10)
                  n190 = case shown="\"结束\"" w394 {
                    selector: w394 -> [w421 w424 w427]
                    tunnel: [w421 w423 w426] -> w390
                    frame Default {
                    }
                    frame "初始化" {
                      n191 = Concatenate Strings("-->>" ("字符串"), w424) -> (w423:string)
                    }
                    frame "结束" {
                      n192 = Concatenate Strings("-->>" ("字符串"), w427) -> (w426:string)
                    }
                  }
                  n193 = global read "VAR总氮全局变量.vi" "状态告警区"() -> (w408:T10)
                  n194 = Insert Into Array(array=w398, new element=w397) -> (w396:string[])  [unwired: 1 in]
                  n195 = Unbundle By Name(w411) -> ("id"=w388:u16)
                  n196 = Unbundle By Name(w393) -> ("工作状态"=w392:T11)
                  n197 = Unbundle By Name(w408) -> ("F0"=w405:sgl, "F1"=w404:sgl, "F2"=w403:sgl, "F3"=w402:sgl, "id"=w401:u16, "flowid"=w400:u16, "量程"=w399:u16)
                  n198 = call "id参数转换.vi"("id"=w388) -> ("table输出"=w387:string)  [unwired: 10 in]
                  n199 = case shown="\"水样测试\"" w392 {
                    tunnel: [_ "【水样测试】" ("字符串") "【标样核查】" ("字符串") "【零点核查】" ("字符串") "【跨度核查】" ("字符串") "【空白测试】" ("字符串") "【平行样测试】" ("字符串") "【加标回收】" ("字符串") "【空白校准】" ("字符串") "【标样校准】" ("字符串")] -> w391
                    frame "空闲", Default {
                    }
                    frame "水样测试" {
                    }
                    frame "标样核查" {
                    }
                    frame "零点核查" {
                    }
                    frame "跨度核查" {
                    }
                    frame "空白测试" {
                    }
                    frame "平行样测试" {
                    }
                    frame "加标回收" {
                    }
                    frame "空白校准" {
                    }
                    frame "标样校准" {
                    }
                  }
                  n200 = Format Into String(format string="F0=%#f,F1=%#f,F2=%#f,F3=%#f,Flow=%d-%-d-%-d" ("格式字符串"), w405, w404, w403, w402, w401, w400, w399) -> (resulting string=w406:string)  [unwired: 2 in, 1 out]
                  n201 = Concatenate Strings(w391, w390) -> (w389:string)
                  n202 = Get Date/Time In Seconds() -> (seconds since 1Jan1904=w409:timestamp)
                  n203 = Bundle By Name(cluster=T21 {"时间标识"=timestamp(0 s since 1904-01-01), "设备"="", "日志信息"="", "流程参数"=""} ("data in"), "时间标识"=w409, "设备"=w387, "日志信息"=w389, "流程参数"=w406) -> (w410:T21)
                  n204 = call "总氮操作日志.vi"("data in"=w410) -> ()  [unwired: 11 in]
                }
              }
            }
            n205 = local write "数组"(w367) -> ()
          }
        }
      }
    }
    n206 = case shown="真" w315 {
      tunnel: w295 -> [_ w452]
      frame False {
      }
      frame True {
        n207 = Subtract(x=w452, y=1) -> (x-y=w450:i32)
        n208 = Subtract(x=w450, y=5) -> (x-y=w454:i32)
        n209 = Greater Or Equal To 0?(x=w454) -> (x >= 0?=w453:bool)
        n210 = property on="多列列表框" class="MCListbox (严格)"() -> (error out=w458:errorcluster, "TopLeft"=w459:T22)  [unwired: 2 in, 1 out]
        n211 = Select(t=w454, s=w453, f=0) -> (s? t:f=w455:i32)
        n212 = Bundle By Name(cluster=w459, "Row"=w455) -> (w460:T22)
        n213 = property on="多列列表框" class="MCListbox (严格)"(error in=w458, "TopLeft"=w460) -> ()  [unwired: 1 in, 2 out]
      }
    }
    n214 = call <vilib>:"Boolean Crossing PtByPt.vi"("input"=w313) -> ("crossing"=w288:bool)  [unwired: 2 in]
    n215 = First Call?() -> (First Call?: T/F=w314:bool)
    n216 = case shown="真" w287 {
      tunnel: w285 -> [_ w338]
      tunnel: w281 -> [_ w342]
      frame False {
      }
      frame True {
        n217 = case shown="\"水样测试\"" w342 {
          tunnel: [_ "【水样测试】" ("字符串") "【标样核查】" ("字符串") "【零点核查】" ("字符串") "【跨度核查】" ("字符串") "【空白测试】" ("字符串") "【平行样测试】" ("字符串") "【加标回收】" ("字符串") "【空白校准】" ("字符串") "【标样校准】" ("字符串")] -> w346
          frame "空闲", Default {
          }
          frame "水样测试" {
          }
          frame "标样核查" {
          }
          frame "零点核查" {
          }
          frame "跨度核查" {
          }
          frame "空白测试" {
          }
          frame "平行样测试" {
          }
          frame "加标回收" {
          }
          frame "空白校准" {
          }
          frame "标样校准" {
          }
        }
        n218 = call "id参数转换.vi"("id"=w338) -> ("table输出"=w339:string)  [unwired: 10 in]
        n219 = Concatenate Strings("-->>" ("字符串"), w346, "启动" ("字符串")) -> (w347:string)
        n220 = Get Date/Time In Seconds() -> (seconds since 1Jan1904=w344:timestamp)
        n221 = Bundle By Name(cluster=T21 {"时间标识"=timestamp(0 s since 1904-01-01), "设备"="", "日志信息"="", "流程参数"=""} ("data in"), "时间标识"=w344, "设备"=w339, "日志信息"=w347) -> (w343:T21)
        n222 = call "总氮操作日志.vi"("data in"=w343) -> ()  [unwired: 11 in]
      }
    }
    n223 = case shown="真" w282 {
      tunnel: w285 -> [_ w319]
      tunnel: w281 -> [_ w323]
      frame False {
      }
      frame True {
        n224 = case shown="\"水样测试\"" w323 {
          tunnel: [_ "【水样测试】" ("字符串") "【标样核查】" ("字符串") "【零点核查】" ("字符串") "【跨度核查】" ("字符串") "【空白测试】" ("字符串") "【平行样测试】" ("字符串") "【加标回收】" ("字符串") "【空白校准】" ("字符串") "【标样校准】" ("字符串")] -> w327
          frame "空闲", Default {
          }
          frame "水样测试" {
          }
          frame "标样核查" {
          }
          frame "零点核查" {
          }
          frame "跨度核查" {
          }
          frame "空白测试" {
          }
          frame "平行样测试" {
          }
          frame "加标回收" {
          }
          frame "空白校准" {
          }
          frame "标样校准" {
          }
        }
        n225 = call "id参数转换.vi"("id"=w319) -> ("table输出"=w320:string)  [unwired: 10 in]
        n226 = Concatenate Strings("-->>" ("字符串"), w327, "停止" ("字符串")) -> (w328:string)
        n227 = Get Date/Time In Seconds() -> (seconds since 1Jan1904=w325:timestamp)
        n228 = Bundle By Name(cluster=T21 {"时间标识"=timestamp(0 s since 1904-01-01), "设备"="", "日志信息"="", "流程参数"=""} ("data in"), "时间标识"=w325, "设备"=w320, "日志信息"=w328) -> (w324:T21)
        n229 = call "总氮操作日志.vi"("data in"=w324) -> ()  [unwired: 11 in]
      }
    }
    n230 = Or(x=w288, y=w314) -> (x .or. y?=w312:bool)
    n231 = Bundle By Name(cluster=T20 {"启动模式"=enum."跨度核查", "启动参数"=1, "量程"=enum."低量程"} ("参数簇"), "启动参数"=w308, "启动模式"=w310, "量程"=w309) -> (w302:T20)
    n232 = while {
      tunnel: w312 -> [w438]
      tunnel: w302 -> [w437]
      shift-right: [w432] -> _
      shift-left: _ -> [w434]
      shift-right: [w433] -> _
      shift-left: _ -> [w435]
      shift-right: ["流程路径"] -> _
      shift-left: _ -> [w431]
      stop <- TRUE stop-if-true
      n233 = Not Equal?(x=w431, y="流程路径") -> (x != y?=w428:bool)
      n234 = Or(x=w438, y=w428) -> (x .or. y?=w429:bool)
      n235 = case shown="真" w429 {
        tunnel: [w440 w448] -> w433
        tunnel: [w439 w447] -> w432
        tunnel: w437 -> [_ w442]
        tunnel: w435 -> [w440 _]
        tunnel: w434 -> [w439 _]
        tunnel: "流程路径" -> [_ w441]
        frame False {
        }
        frame True {
          n236 = call "斯坦道XML解析.vi"("添加的路径"=w441, "参数簇"=w442) -> ("步骤时间"=w443:string[], "步骤名"=w445:string[])  [unwired: 8 in]
          n237 = Build Array(w445, w443) -> (w444:string[][])
          n238 = for {
            tunnel: w445 -> [_] mode=indexing
            tunnel: [w449] -> w446 mode=indexing
            i -> [w449]
          }
          n239 = Transpose 2D Array(2D array=w444) -> (transposed array=w447:string[][])
          n240 = Number To Decimal String(number=w446) -> (decimal integer string=w448:string[])  [unwired: 1 in]
        }
      }
      n241 = property on="多列列表框" class="MCListbox (严格)"("ItemNames"=w432, "RowHdrs[]"=w433) -> ()  [unwired: 2 in, 2 out]
    }
    n242 = Wait (ms)(milliseconds to wait=u32 1000 ("等待时间（毫秒）")) -> ()  [unwired: 1 out]
  }
  n243 = Bundle("参数下拉列表"=w12, "测量模式下拉列表"=w11, "量程下拉列表"=w10) -> (w9:T23)  [unwired: 1 in]
  n244 = property on="曲线模型" class="曲线模型 (严格)"("属性"=w9) -> (error out=w17:errorcluster)  [unwired: 2 in, 1 out]
  n245 = control-ref of="量程参数读取"() -> (w13:refnum<vi>)
  n246 = control-ref of="公式"() -> (w22:refnum<vi>)
  n247 = control-ref of="参数下拉列表"() -> (w24:refnum<vi>)
  n248 = control-ref of="测量模式下拉列表"() -> (w23:refnum<vi>)
  n249 = control-ref of="量程下拉列表"() -> (w25:refnum<vi>)
  n250 = Obtain Notifier(name (unnamed)="TN" ("名称（未命名）"), notification data type=FALSE) -> (notifier out=w14:refnum<notifier>)  [unwired: 2 in, 2 out]
  n251 = Obtain Queue(name (unnamed)="TN" ("名称（未命名）"), element data type=cluster{"命令":string, "data":variant} {"命令"="", "data"=variant}) -> (queue out=w26:refnum<queue>, error out=w27:errorcluster)  [unwired: 3 in, 1 out]
  n252 = while {
    tunnel: w26 -> [w466]
    tunnel: w27 -> [_]
    stop <- FALSE stop-if-true
    n253 = Get Queue Status(queue=w466) -> (queue out=w462:refnum<queue>, # elements in queue=w461:i32)  [unwired: 2 in, 6 out]
    n254 = global read "总氮断电保存全局变量.vi" "流程路径"() -> (w465:path)
    n255 = global read "总氮断电保存全局变量.vi" "MB通信方式选择"() -> (w463:enum16{"串口", "TCP"})
    n256 = case shown="0" w461 {
      tunnel: w462 -> [_ w472]
      frame Default {
      }
      frame 0 {
        w481 = u16 2 items=["总磷"=1, "总氮"=2, "氨氮"=3] ("站号")
        # "试剂填充 172 \n管路清洗108\n氨氮92\n总磷131\n总磷海水147\n总氮76\n总氮海水92"
        n257 = global read "VAR总氮全局变量.vi" "状态告警区"() -> (w473:T10)
        n258 = Unbundle By Name(w473) -> ("系统时间"=w480:timestamp, "工作状态"=w471:T11)
        n259 = Bundle By Name(cluster=cluster{"命令":string, "data":variant} {"命令"="", "data"=variant} ("元素"), "命令"="读状态告警区", "data"=w481) -> (w484:cluster{"命令":string, "data":variant})
        n260 = Get Date/Time In Seconds() -> (seconds since 1Jan1904=w479:timestamp)
        n261 = Enqueue Element(queue=w472, element=w484) -> (queue out=w482:refnum<queue>)  [unwired: 2 in, 2 out]
        n262 = Subtract(x=w479, y=w480) -> (x-y=w478:dbl)
        n263 = Equal?(x=w471, y=T11."空闲") -> (x = y?=w469:bool)
        n264 = Absolute Value(x=w478) -> (abs(x)=w477:dbl)
        n265 = case shown="真" w469 {
          tunnel: w482 -> [w486 w489]
          tunnel: w481 -> [_ w488]
          tunnel: [w486 w487] -> w474
          frame False {
          }
          frame True {
            n266 = Bundle By Name(cluster=cluster{"命令":string, "data":variant} {"命令"="", "data"=variant} ("元素"), "命令"="读测量数据区", "data"=w488) -> (w491:cluster{"命令":string, "data":variant})
            n267 = Enqueue Element(queue=w489, element=w491) -> (queue out=w487:refnum<queue>)  [unwired: 2 in, 2 out]
          }
        }
        n268 = Greater Or Equal?(x=w477, y=120.0) -> (x >= y?=w475:bool)
        n269 = case shown="真" w475 {
          tunnel: w474 -> [_ w494]
          frame False {
          }
          frame True {
            n270 = call "总氮启动命令.vi"("参数"=T24 {"站号"=3, "量程切换"=enum."AUTO", "控制命令"=enum."校时", "模式设置"=enum."待机", "测量间隔"=0}) -> ("启动命令"=w493:cluster{"命令":string, "data":variant})  [unwired: 10 in]
            n271 = Enqueue Element(queue=w494, element=w493) -> ()  [unwired: 2 in, 3 out]
          }
        }
      }
    }
    n272 = local write "流程路径"(w465) -> ()
    n273 = case shown="\"TCP\"" w463 {
      tunnel: [w496 w497] -> w464
      frame "串口", Default {
        n274 = global read "总氮断电保存全局变量.vi" "VISA Resource"() -> (w496:refnum<visa-resource-name>)
      }
      frame "TCP" {
        n275 = global read "总氮断电保存全局变量.vi" "IP"() -> (w497:string)
      }
    }
    "字符串" <- w464
    n276 = Wait (ms)(milliseconds to wait=u32 1000 ("等待时间（毫秒）")) -> ()  [unwired: 1 out]
  }
  n277 = while {
    tunnel: w26 -> [w504]
    tunnel: w25 -> [w503]
    tunnel: w24 -> [w502]
    tunnel: w23 -> [w501]
    tunnel: w22 -> [w500]
    tunnel: w13 -> [w499]
    tunnel: w17 -> [_]
    tunnel: w14 -> [w498]
    stop <- FALSE stop-if-true
    n278 = event shown="[16] \"设置\": 值改变" {
      selector: _ -> [_ _ _ _ _ _ _ _ _ _ _ _ _ _ _ _ _ _ _ _ _ _ _]
      dyn-events: _ -> [_ _ _ _ _ _ _ _ _ _ _ _ _ _ _ _ _ _ _ _ _ _ _]
      timeout: _ -> [_ _ _ _ _ _ _ _ _ _ _ _ _ _ _ _ _ _ _ _ _ _ _]
      tunnel: w504 -> [_ _ _ _ w532 w546 _ _ _ _ _ _ w606 _ w616 w651 _ _ _ _ _ _ _]
      tunnel: w503 -> [_ _ _ w510 _ _ _ _ _ _ _ _ _ _ _ _ w661 _ _ w684 w687 _ _]
      tunnel: w502 -> [_ _ _ w512 _ _ _ _ _ _ _ _ _ _ _ _ w663 _ _ w682 w689 w739 w746]
      tunnel: w501 -> [_ _ _ w511 _ _ _ _ _ _ _ _ _ _ _ _ w662 _ _ w683 w688 _ _]
      tunnel: w500 -> [_ _ _ w513 _ _ _ _ _ _ _ _ _ _ _ _ w664 _ _ w678 _ _ _]
      tunnel: w499 -> [_ _ _ _ _ _ _ _ _ _ _ _ _ _ _ _ w658 _ _ _ _ w737 _]
      tunnel: w498 -> [_ _ _ _ _ _ _ _ _ _ _ _ _ _ _ w647 _ _ _ _ _ _ _]
      tunnel: [_ _ _ w518 _ _ _ _ _ _ _ _ _ _ _ _ _ _ _ _ _ _ _] -> _
      tunnel: [_ _ _ _ _ _ _ _ _ _ _ _ _ _ _ _ w652 _ _ _ _ _ _] -> _
      event Timeout {
        n279 = event-data() -> ()  [unwired: 1 in, 3 out]
      }
      event "流程固件": Value Change {
        # "试剂填充 172 \n管路清洗108\n氨氮92\n总磷131\n总磷海水147\n总氮76\n总氮海水92"
        n280 = event-data() -> ()  [unwired: 1 in, 6 out]
        n281 = call "流程固件设置对话框.vi"() -> ()  [unwired: 12 in]
      }
      event "布尔": Mouse Down {
        n282 = event-data() -> ("CtlRef"=w507:refnum<vi>)  [unwired: 1 in, 5 out]
        n283 = property class="Bool (严格)"(reference=w507) -> ("Value"=w506:bool)  [unwired: 1 in, 2 out]
        n284 = case shown="假" w506 {
          frame False {
            n285 = call "密码键盘.vi"() -> ("NewNumber"=→"输入密码":dbl)  [unwired: 1 in]
          }
          frame True {
            n286 = local write "输入密码"(u32 0 ("输入密码")) -> ()
          }
        }
      }
      event "测量模式下拉列表", "量程下拉列表", "参数下拉列表": Value Change {
        n287 = event-data() -> ()  [unwired: 1 in, 6 out]
        n288 = property class="Enum (严格)"(reference=w512) -> ("Value"=w517:enum16{"总磷", "总氮"})  [unwired: 1 in, 2 out]
        n289 = property class="Enum (严格)"(reference=w511) -> ("Value"=w516:enum16{"水样测量", "零点核查", "跨度核查", "标样核查", "加标回收"})  [unwired: 1 in, 2 out]
        n290 = property class="Enum (严格)"(reference=w510) -> ("Value"=w515:enum16{"低量程", "高量程"})  [unwired: 1 in, 2 out]
        n291 = call "总磷总氮公式读取.vi"("量程"=w515, "测量模式"=w516, "测量参数"=w517) -> ("公式"=w514:cluster{"X^2":dbl, "X":dbl, "b":dbl})  [unwired: 7 in, 1 out]
        n292 = property class="Clust (严格)"(reference=w513, "Value"=w514) -> ()  [unwired: 1 in, 2 out]
        n293 = local read "参数下拉列表"() -> (w519:enum16{"总磷", "总氮"})
        n294 = local read "测量模式下拉列表"() -> (w520:enum16{"水样测量", "零点核查", "跨度核查", "标样核查", "加标回收"})
        n295 = local read "量程下拉列表"() -> (w521:enum16{"低量程", "高量程"})
        n296 = Bundle("参数下拉列表"=w519, "测量模式下拉列表"=w520, "量程下拉列表"=w521) -> (w522:T23)  [unwired: 1 in]
        n297 = property on="曲线模型" class="曲线模型 (严格)"("属性"=w522) -> (error out=w518:errorcluster)  [unwired: 2 in, 1 out]
      }
      event "串口设置": Value Change {
        n298 = event-data() -> ()  [unwired: 1 in, 6 out]
        n299 = global read "总氮断电保存全局变量.vi" "VISA Resource"() -> (w529:refnum<visa-resource-name>)
        n300 = global read "总氮断电保存全局变量.vi" "MB通信方式选择"() -> (w523:enum16{"串口", "TCP"})
        n301 = global read "总氮断电保存全局变量.vi" "IP"() -> (w524:string)
        n302 = global read "总氮断电保存全局变量.vi" "PORT"() -> (w528:string)
        n303 = call "串口配置.vi"("PORT"=w528, "IP"=w524, "MB通信方式选择"=w523, "请选择串口:"=w529) -> ("PORT 2"=w526:string, "IP 2"=w527:string, "确认 2"=w530:bool, "VISA资源名称 2"=w531:refnum<visa-resource-name>, "MB通信方式选择 2"=w525:enum16{"串口", "TCP"})  [unwired: 3 in]
        n304 = case shown="真" w530 {
          tunnel: w531 -> [_ w537]
          tunnel: w532 -> [_ w536]
          tunnel: w527 -> [_ w535]
          tunnel: w526 -> [_ w534]
          tunnel: w525 -> [_ w533]
          frame False {
          }
          frame True {
            n305 = flat-sequence {
              tunnel: w537 -> [w542]
              tunnel: w536 -> [w543]
              tunnel: w535 -> [w541]
              tunnel: w534 -> [w540]
              tunnel: w533 -> [w539]
              frame #0 {
                n306 = global write "总氮断电保存全局变量.vi" "IP"(w541) -> ()
                n307 = global write "总氮断电保存全局变量.vi" "PORT"(w540) -> ()
                n308 = global write "总氮断电保存全局变量.vi" "MB通信方式选择"(w539) -> ()
                n309 = global write "总氮断电保存全局变量.vi" "VISA Resource"(w542) -> ()
                n310 = Flush Queue(queue=w543) -> (queue out=w538:refnum<queue>)  [unwired: 1 in, 2 out]
                n311 = Enqueue Element(queue=w538, element=cluster{"命令":string, "data":variant} {"命令"="启用模块", "data"=variant} ("元素")) -> ()  [unwired: 2 in, 3 out]
              }
              frame #1 {
                n312 = call "配置文件保存.vi"() -> ()  [unwired: 12 in]
              }
            }
          }
        }
      }
      event "模块启用": Value Change {
        n313 = event-data() -> ("OldVal"=w547:bool)  [unwired: 1 in, 5 out]
        n314 = Flush Queue(queue=w546) -> (queue out=w545:refnum<queue>)  [unwired: 1 in, 2 out]
        n315 = case shown="假" w547 {
          tunnel: w545 -> [w548 w550]
          frame False {
            n316 = Enqueue Element(queue=w548, element=cluster{"命令":string, "data":variant} {"命令"="停用模块", "data"=variant} ("元素")) -> ()  [unwired: 2 in, 3 out]
          }
          frame True {
            n317 = Enqueue Element(queue=w550, element=cluster{"命令":string, "data":variant} {"命令"="启用模块", "data"=variant} ("元素")) -> ()  [unwired: 2 in, 3 out]
          }
        }
      }
      event "流程路径": Value Change {
        n318 = event-data() -> ()  [unwired: 1 in, 6 out]
        n319 = flat-sequence {
          frame #0 {
            n320 = local read "流程路径"() -> (w552:path)
            n321 = global write "总氮断电保存全局变量.vi" "流程路径"(w552) -> ()
          }
          frame #1 {
            n322 = call "配置文件保存.vi"() -> ()  [unwired: 12 in]
          }
        }
      }
      event "公式一键写入": Value Change {
        n323 = event-data() -> ()  [unwired: 1 in, 6 out]
        n324 = local read "公式"() -> (w553:cluster{"X^2":dbl, "X":dbl, "b":dbl})
        n325 = call "公式复合写入.vi"("公式"=w553) -> ()  [unwired: 11 in]
      }
      event "曲线模型": Value Change {
        n326 = event-data() -> ()  [unwired: 1 in, 6 out]
        n327 = disable-structure shown="禁用" {
          frame Disabled {
            n328 = Unbundle By Name("曲线模型") -> ("X^2"=w556:dbl, "X"=w557:dbl, "B"=w558:dbl)
            n329 = Build Array(w556, w557, w558) -> (w555:dbl[])
            n330 = Array To Cluster(array=w555) -> (cluster=w554:cluster{"[0]":dbl, "[1]":dbl, "[2]":dbl})
            n331 = local write "公式"(w554) -> ()
          }
          frame Enabled {
          }
        }
      }
      event "质控参数设置": Value Change {
        n332 = event-data() -> ()  [unwired: 1 in, 6 out]
        n333 = global read "总氮断电保存全局变量.vi" "质控参数设置"() -> (w560:T25)
        n334 = call "总氮质控参数设置.vi"("质控参数设置"=w560) -> ("输出簇"=w561:T26)  [unwired: 10 in]
        n335 = Unbundle By Name(w561) -> ("确定"=w562:bool)
        n336 = case shown="真" w562 {
          tunnel: w561 -> [_ w564]
          tunnel: w560 -> [_ w563]
          frame False {
          }
          frame True {
            n337 = flat-sequence {
              tunnel: w564 -> [w571]
              tunnel: w563 -> [w570]
              frame #0 {
                n338 = Unbundle By Name(w571) -> ("跨度值"=w569:dbl, "零点标准液浓度"=w568:dbl, "跨度标准液浓度"=w567:dbl, "标准液标准浓度"=w566:dbl)
                n339 = Bundle By Name(cluster=w570, "跨度值"=w569, "零点标准液浓度"=w568, "跨度标准液浓度"=w567, "标准液标准浓度"=w566) -> (w565:T25)
                n340 = global write "总氮断电保存全局变量.vi" "质控参数设置"(w565) -> ()
              }
              frame #1 {
                n341 = call "配置文件保存.vi"() -> ()  [unwired: 12 in]
              }
            }
          }
        }
      }
      event "仪器参数设置": Value Change {
        n342 = event-data() -> ()  [unwired: 1 in, 6 out]
        n343 = global read "总氮断电保存全局变量.vi" "总氮仪器参数"() -> (w572:T27)
        n344 = call "仪器参数设置.vi"("氨氮仪器参数"=w572) -> ("仪器参数设置输出"=w573:T28)  [unwired: 10 in]
        n345 = Unbundle By Name(w573) -> ("确定"=w574:bool)
        n346 = case shown="真" w574 {
          tunnel: w573 -> [_ w576]
          tunnel: w572 -> [_ w575]
          frame False {
          }
          frame True {
            n347 = flat-sequence {
              tunnel: w576 -> [w593]
              tunnel: w575 -> [w592]
              frame #0 {
                n348 = Unbundle By Name(w593) -> ("测量量程"=w591:dbl, "测量精度"=w590:dbl, "测量间隔"=w589:dbl, "消解温度"=w588:dbl, "消解时长"=w586:dbl, "空白校准时间"=w585:timestamp, "曲线截距"=w584:dbl, "曲线斜率"=w583:dbl, "测量检出限"=w582:dbl, "测量信号值"=w581:dbl, "线性相关系数"=w580:dbl, "二次多项式系数"=w579:dbl, "标样校准时间"=w578:timestamp, "稀释倍数"=w577:dbl)
                n349 = Bundle By Name(cluster=w592, "测量量程"=w591, "测量精度"=w590, "测量间隔"=w589, "消解温度"=w588, "消解时长"=w586, "空白校准时间"=w585, "曲线截距"=w584, "曲线斜率"=w583, "测量检出限"=w582, "测量信号值"=w581, "线性相关系数"=w580, "二次多项式系数"=w579, "标样校准时间"=w578, "稀释倍数"=w577) -> (w587:T27)
                n350 = global write "总氮断电保存全局变量.vi" "总氮仪器参数"(w587) -> ()
              }
              frame #1 {
                n351 = call "配置文件保存.vi"() -> ()  [unwired: 12 in]
              }
            }
          }
        }
      }
      event "自动测试量程配置": Value Change {
        n352 = event-data() -> ()  [unwired: 1 in, 6 out]
        n353 = flat-sequence {
          frame #0 {
            n354 = global write "总氮断电保存全局变量.vi" "总氮自动测试量程配置"("自动测试量程配置") -> ()
          }
          frame #1 {
            n355 = call "配置文件保存.vi"() -> ()  [unwired: 12 in]
          }
        }
      }
      event "手动启动": Value Change {
        n356 = event-data() -> ()  [unwired: 1 in, 6 out]
        n357 = call "总氮启动参数对话框.vi"() -> ("标样浓度输出"=w595:dbl, "确认"=w605:bool, "元素"=w597:cluster{"命令":string, "data":variant})  [unwired: 9 in]
        n358 = case shown="真" w605 {
          tunnel: w606 -> [_ w612]
          tunnel: w597 -> [_ w611]
          frame False {
          }
          frame True {
            n359 = Enqueue Element(queue=w612, element=w611) -> ()  [unwired: 2 in, 3 out]
          }
        }
        n360 = Unbundle By Name(w597) -> ("data"=w603:variant)
        n361 = Variant To Data(type=cluster{"站号":u16, "控制命令":u16[]} {"站号"=0, "控制命令"=[]} ("输出簇"), Variant=w603) -> (data=w602:cluster{"站号":u16, "控制命令":u16[]})  [unwired: 1 in, 1 out]
        n362 = Unbundle By Name(w602) -> ("控制命令"=w601:u16[])
        n363 = Index Array(array=w601) -> (element=w600:u16)  [unwired: 1 in]
        n364 = Swap Bytes(anything=w600) -> (byte swapped=w599:u16)
        n365 = Equal?(x=w599, y=u16 2) -> (x = y?=w596:bool)
        n366 = case shown="真" w596 {
          tunnel: w595 -> [_ w607]
          frame False {
          }
          frame True {
            n367 = flat-sequence {
              tunnel: w607 -> [w609]
              frame #0 {
                n368 = global read "总氮断电保存全局变量.vi" "质控参数设置"() -> (w610:T25)
                n369 = Bundle By Name(cluster=w610, "标准液标准浓度"=w609) -> (w608:T25)
                n370 = global write "总氮断电保存全局变量.vi" "质控参数设置"(w608) -> ()
              }
              frame #1 {
                n371 = call "配置文件保存.vi"() -> ()  [unwired: 12 in]
              }
            }
          }
        }
      }
      event "单步测试": Value Change {
        n372 = event-data() -> ()  [unwired: 1 in, 6 out]
        n373 = call "总氮单步调试对话框.vi"() -> ()  [unwired: 12 in]
      }
      event "校准按钮.校准1", "校准按钮.校准2", "校准按钮.校准3", "校准按钮.校准4", "校准按钮.校准5": Value Change {
        n374 = event-data() -> ("CtlRef"=w622:refnum<vi>)  [unwired: 1 in, 5 out]
        n375 = property class="Bool"(reference=w622) -> ("Label.Text"=w620:string)  [unwired: 1 in, 2 out]
        n376 = property on="曲线模型" class="曲线模型 (严格)"() -> ("浓度属性"=w621:T29)  [unwired: 2 in, 2 out]
        n377 = case shown="\"校准3\"" w620 {
          tunnel: [w630 w633 w636 w639 w642] -> w618
          tunnel: [u16 1 ("校准点1-5") u16 2 ("校准点1-5") u16 3 ("校准点1-5") u16 4 ("校准点1-5") u16 5 ("校准点1-5")] -> w619
          tunnel: w621 -> [w631 w634 w637 w640 w643]
          frame "校准1", Default {
            n378 = Unbundle By Name(w631) -> ("标液浓度1"=w630:dbl)
          }
          frame "校准2" {
            n379 = Unbundle By Name(w634) -> ("标液浓度2"=w633:dbl)
          }
          frame "校准3" {
            n380 = Unbundle By Name(w637) -> ("标液浓度3"=w636:dbl)
          }
          frame "校准4" {
            n381 = Unbundle By Name(w640) -> ("标液浓度4"=w639:dbl)
          }
          frame "校准5" {
            n382 = Unbundle By Name(w643) -> ("标液浓度5"=w642:dbl)
          }
        }
        n383 = Not Equal To 0?(x=w618) -> (x != 0?=w614:bool)
        n384 = Bundle By Name(cluster=cluster{"校准？":bool, "校准点1-5":u16, "校准浓度":dbl} {"校准？"=FALSE, "校准点1-5"=0, "校准浓度"=0.0} ("校准输出"), "校准？"=TRUE, "校准点1-5"=w619, "校准浓度"=w618) -> (w617:cluster{"校准？":bool, "校准点1-5":u16, "校准浓度":dbl})
        n385 = global write "总氮断电保存全局变量.vi" "校准输出"(w617) -> ()
        n386 = local read "量程下拉列表"() -> (w613:enum16{"低量程", "高量程"})
        n387 = case shown="真" w614 {
          tunnel: [cluster{"命令":string, "data":variant} {"命令"="启动", "data"=variant(cluster{"站号":u16, "控制命令":u16[]} {"站号"=2, "控制命令"=[2048, 256]})} ("元素") w626] -> w615
          tunnel: w613 -> [_ w627]
          frame False {
            # "校零"
          }
          frame True {
            # "校标"
            n388 = case shown="\"低量程\", 默认" w627 {
              tunnel: [cluster{"命令":string, "data":variant} {"命令"="启动", "data"=variant(cluster{"站号":u16, "控制命令":u16[]} {"站号"=2, "控制命令"=[2304, 256]})} ("元素") cluster{"命令":string, "data":variant} {"命令"="启动", "data"=variant(cluster{"站号":u16, "控制命令":u16[]} {"站号"=2, "控制命令"=[2304, 257]})} ("元素")] -> w626
              frame "低量程", Default {
              }
              frame "高量程" {
              }
            }
          }
        }
        n389 = Enqueue Element(queue=w616, element=w615) -> ()  [unwired: 2 in, 3 out]
      }
      event "停止": Value Change {
        n390 = event-data() -> ()  [unwired: 1 in, 6 out]
        n391 = Cancel Notification(0:w647) -> (8:w646:refnum<notifier>)  [unwired: 1 in, 2 out]
        n392 = Enqueue Element(queue=w651, element=cluster{"命令":string, "data":variant} {"命令"="启动", "data"=variant(cluster{"站号":u16, "控制命令输出":u16[]} {"站号"=1, "控制命令输出"=[2816]})} ("元素")) -> (queue out=w648:refnum<queue>)  [unwired: 2 in, 2 out]
        n393 = Send Notification(notification=TRUE ("通知"), notifier=w646) -> ()  [unwired: 1 in, 2 out]
        n394 = Enqueue Element(queue=w648, element=cluster{"命令":string, "data":variant} {"命令"="启动", "data"=variant(cluster{"站号":u16, "控制命令输出":u16[]} {"站号"=2, "控制命令输出"=[2816]})} ("元素")) -> ()  [unwired: 2 in, 3 out]
      }
      event "设置": Value Change {
        n395 = event-data() -> ()  [unwired: 1 in, 6 out]
        n396 = property class="Enum (严格)"(reference=w663) -> (reference out=w657:refnum<vi>, "Value"=w668:enum16{"总磷", "总氮"})  [unwired: 1 in, 1 out]
        n397 = property class="Enum (严格)"(reference=w662) -> ("Value"=w667:enum16{"水样测量", "零点核查", "跨度核查", "标样核查", "加标回收"})  [unwired: 1 in, 2 out]
        n398 = property class="Enum (严格)"(reference=w661) -> ("Value"=w666:enum16{"低量程", "高量程"})  [unwired: 1 in, 2 out]
        n399 = property on="窗格" class="Pane"("Origin"=T8 {"Horizontal"=0, "Vertical"=628} ("原点")) -> ()  [unwired: 2 in, 2 out]
        n400 = call "总磷总氮公式读取.vi"("量程"=w666, "测量模式"=w667, "测量参数"=w668) -> ("error out"=w656:errorcluster, "公式"=w665:cluster{"X^2":dbl, "X":dbl, "b":dbl})  [unwired: 7 in]
        n401 = property class="Clust (严格)"(reference=w664, error in=w656, "Value"=w665) -> (error out=w655:errorcluster)  [unwired: 1 out]
        n402 = property class="Enum (严格)"(reference=w657, error in=w655) -> (error out=w654:errorcluster, "Value"=w660:enum16{"总磷", "总氮"})  [unwired: 1 out]
        n403 = call "总磷总氮量程读取.vi"("error in (no error)"=w654, "测量参数"=w660) -> ("error out"=w653:errorcluster, "量程参数读取"=w659:T30)  [unwired: 8 in]
        n404 = property class="Clust (严格)"(reference=w658, error in=w653, "Value"=w659) -> (error out=w652:errorcluster)  [unwired: 1 out]
      }
      event "返回": Value Change {
        n405 = event-data() -> ()  [unwired: 1 in, 6 out]
        n406 = property on="窗格" class="Pane"("Origin"=T8 {"Horizontal"=0, "Vertical"=0} ("原点")) -> ()  [unwired: 2 in, 2 out]
      }
      event "公式.X^2", "公式.X", "公式.b", "量程参数读取.测量精度", "量程参数读取.检出限", "量程参数读取.上限", "量程参数读取.下限", "量程参数读取.(低->高)", "量程参数读取.(高->低)", "量程参数读取.稀释度": Mouse Down {
        n407 = event-data() -> ("CtlRef"=w674:refnum<vi>)  [unwired: 1 in, 5 out]
        n408 = property class="DigNum (严格)"(reference=w674) -> (reference out=w672:refnum<vi>, "Value"=w673:dbl)  [unwired: 1 in, 1 out]
        n409 = call "数字键盘.vi"("OldNumber"=w673) -> ("NewNumber"=w671:dbl)
        n410 = property class="DigNum (严格)"(reference=w672, "Val(Sgnl)"=w671) -> ()  [unwired: 1 in, 2 out]
      }
      event "读公式": Value Change {
        n411 = event-data() -> ()  [unwired: 1 in, 6 out]
        n412 = property class="Enum (严格)"(reference=w682) -> ("Value"=w681:enum16{"总磷", "总氮"})  [unwired: 1 in, 2 out]
        n413 = property class="Enum (严格)"(reference=w683) -> ("Value"=w680:enum16{"水样测量", "零点核查", "跨度核查", "标样核查", "加标回收"})  [unwired: 1 in, 2 out]
        n414 = property class="Enum (严格)"(reference=w684) -> ("Value"=w679:enum16{"低量程", "高量程"})  [unwired: 1 in, 2 out]
        n415 = call "总磷总氮公式读取.vi"("量程"=w679, "测量模式"=w680, "测量参数"=w681) -> ("error out"=w676:errorcluster, "公式"=w677:cluster{"X^2":dbl, "X":dbl, "b":dbl})  [unwired: 7 in]
        n416 = property class="Clust (严格)"(reference=w678, "Value"=w677) -> ()  [unwired: 1 in, 2 out]
        n417 = case shown="错误" w676 {
          tunnel: ["读取成功" ("消息") "读取失败" ("消息")] -> w675
          frame No Error {
          }
          frame Error {
          }
        }
        n418 = One Button Dialog(message=w675) -> ()  [unwired: 1 in, 1 out]
      }
      event "写公式": Value Change {
        n419 = event-data() -> ()  [unwired: 1 in, 6 out]
        n420 = call <vilib>:"Three Button Dialog.vi"("Allow user to close window? (TRUE)"=FALSE, "Center Button Text (\"No\")"="一键写入所有公式" ("F按钮名称（“取消”）"), "Left Button Text (\"Yes\")"="写入当前公式" ("T按钮名称（“确定”）"), "message"="即将将左侧拟合公式写入仪器\n请选择写入当前模式和量程还是一键写入所有模式量程！" ("消息")) -> ("Which Button?"=w690:T31)  [unwired: 7 in]
        n421 = case shown="\"Left Button\", 默认" w690 {
          tunnel: w689 -> [w697 w727 _ _]
          tunnel: w688 -> [w696 w726 _ _]
          tunnel: w687 -> [w695 w725 _ _]
          frame "Left Button", Default {
            n422 = local read "曲线模型"() -> (w703:cluster{"X^2":dbl, "X":dbl, "B":dbl, "r^2":dbl})
            n423 = Unbundle By Name(w703) -> ("X^2"=w701:dbl, "X"=w700:dbl, "B"=w699:dbl)
            n424 = Build Array(w701, w700, w699) -> (w702:dbl[])
            n425 = Array To Cluster(array=w702) -> (cluster=w698:cluster{"[0]":dbl, "[1]":dbl, "[2]":dbl})
            n426 = call "总磷总氮公式写入.vi"("公式"=w698, "量程"="量程下拉列表", "测量模式"="测量模式下拉列表", "测量参数"="参数下拉列表") -> ("error out"=w707:errorcluster)  [unwired: 7 in]
            n427 = call "公式发生改变存储 (子VI).vi"("公式"=w698, "量程下拉列表输入"=w695, "测量模式下拉列表输入"=w696, "参数"=w697) -> ()  [unwired: 8 in]
            n428 = local write "公式"(w698) -> ()
            n429 = case shown="无错误" w707 {
              tunnel: ["写入成功" ("消息") "写入失败" ("消息")] -> w708
              tunnel: "测量模式下拉列表" -> [w711 _]
              tunnel: "量程下拉列表" -> [w710 _]
              tunnel: w698 -> [w709 _]
              frame No Error {
                n430 = Equal?(x=w711, y=enum16{"水样测量", "零点核查", "跨度核查", "标样核查", "加标回收"}."水样测量") -> (x = y?=w714:bool)
                n431 = Equal?(x=w710, y=enum16{"低量程", "高量程"}."低量程") -> (x = y?=w713:bool)
                n432 = Compound Arithmetic op=AND ("复合运算")(w714, w713) -> (w712:bool)
                n433 = case shown="真" w712 {
                  tunnel: w709 -> [_ w723]
                  frame False {
                  }
                  frame True {
                    n434 = Unbundle By Name(w723) -> ("[0]"=w720:dbl, "[1]"=w722:dbl, "[2]"=w721:dbl)
                    n435 = global read "总氮断电保存全局变量.vi" "总氮仪器参数"() -> (w719:T27)
                    n436 = Bundle By Name(cluster=w719, "曲线截距"=w721, "曲线斜率"=w722, "二次多项式系数"=w720) -> (w718:T27)
                    n437 = global write "总氮断电保存全局变量.vi" "总氮仪器参数"(w718) -> ()
                  }
                }
              }
              frame Error {
              }
            }
            n438 = One Button Dialog(message=w708) -> ()  [unwired: 1 in, 1 out]
          }
          frame "Center Button" {
            n439 = local read "曲线模型"() -> (w733:cluster{"X^2":dbl, "X":dbl, "B":dbl, "r^2":dbl})
            n440 = Unbundle By Name(w733) -> ("X^2"=w731:dbl, "X"=w730:dbl, "B"=w729:dbl)
            n441 = Build Array(w731, w730, w729) -> (w732:dbl[])
            n442 = Array To Cluster(array=w732) -> (cluster=w728:cluster{"[0]":dbl, "[1]":dbl, "[2]":dbl})
            n443 = local write "公式"(w728) -> ()
            n444 = call "公式复合写入.vi"("公式"=w728) -> ()  [unwired: 11 in]
            n445 = call "公式发生改变存储 (子VI).vi"("公式"=w728, "量程下拉列表输入"=w725, "测量模式下拉列表输入"=w726, "参数"=w727) -> ()  [unwired: 8 in]
          }
          frame "Right Button" {
          }
          frame "Window Close" {
          }
        }
      }
      event "量程切换阈值读取": Value Change {
        n446 = event-data() -> ()  [unwired: 1 in, 6 out]
        n447 = property class="Enum (严格)"(reference=w739) -> ("Value"=w738:enum16{"总磷", "总氮"})  [unwired: 1 in, 2 out]
        n448 = call "总磷总氮量程读取.vi"("测量参数"=w738) -> ("error out"=w734:errorcluster, "量程参数读取"=w736:T30)  [unwired: 9 in]
        n449 = property class="Clust (严格)"(reference=w737, "Value"=w736) -> ()  [unwired: 1 in, 2 out]
        n450 = case shown="错误" w734 {
          tunnel: ["读取成功" ("消息") "读取失败" ("消息")] -> w735
          frame No Error {
          }
          frame Error {
          }
        }
        n451 = One Button Dialog(message=w735) -> ()  [unwired: 1 in, 1 out]
      }
      event "量程切换阈值写入": Value Change {
        n452 = event-data() -> ()  [unwired: 1 in, 6 out]
        n453 = property class="Enum (严格)"(reference=w746) -> ("Value"=w745:enum16{"总磷", "总氮"})  [unwired: 1 in, 2 out]
        n454 = call "总磷总氮量程写入.vi"("量程参数写入"="量程参数读取", "测量参数"=w745) -> ("error out"=w743:errorcluster)  [unwired: 8 in]
        n455 = case shown="无错误" w743 {
          tunnel: ["写入成功" ("消息") "写入失败" ("消息")] -> w744
          frame No Error {
          }
          frame Error {
          }
        }
        n456 = One Button Dialog(message=w744) -> ()  [unwired: 1 in, 1 out]
      }
    }
  }
  n457 = while {
    tunnel: [w756] -> _
    shift-right: [w754] -> _
    shift-left: w7 -> [w753]
    tunnel: w4 -> [w750]
    stop <- FALSE stop-if-true
    n458 = global read "VAR总氮全局变量.vi" "配置文件 path"() -> (w749:path)
    n459 = Read from Text File(file (use dialog)=w749, error in=w750) -> (text=w754:string, error out=w751:errorcluster)  [unwired: 2 in, 2 out]
    n460 = Not Equal?(x=w754, y=w753) -> (x != y?=w752:bool)
    n461 = case shown="真" w752 {
      tunnel: [w758 w762] -> w756
      tunnel: w749 -> [_ w761]
      tunnel: w751 -> [w758 w760]
      frame False {
      }
      frame True {
        # "文件发生改变进行更新"
        n462 = call <vilib>:"Open Config Data.vi"("error in (no error)"=w760, "configuration file path"=w761) -> ("error out"=w766:errorcluster, "refnum"=w765:T13)  [unwired: 7 in, 1 out]
        n463 = vi-ref "总氮断电保存全局变量.vi"() -> (w759:refnum<vi>)
        n464 = call <userlib>:"Read Panel from INI__ogtk.vi"("error in (no error)"=w766, "VI ref"=w759, "refnum"=w765) -> ("error out"=w764:errorcluster, "refnum out"=w763:T13)  [unwired: 7 in]
        n465 = call <vilib>:"Close Config Data.vi"("error in (no error)"=w764, "refnum"=w763) -> ("error out"=w762:errorcluster)  [unwired: 8 in, 1 out]
      }
    }
    n466 = Wait (ms)(milliseconds to wait=u32 1000 ("等待时间（毫秒）")) -> ()  [unwired: 1 out]
  }
